vi "Main.vi"() -> ()   [LabVIEW 2014]
uses:
  vis/Controls/OtherSpec.ctl
  <vilib>/userdefined/High Color/IMAQdx.ctl
  vis/ModelEditSubVIs/ModeEditeControl.ctl
  vis/ModelEditSubVIs/ModelInfo.ctl
  vis/Controls/XYPos.ctl
  vis/Controls/MsgAction.ctl
  vis/SaveTestDataSubVI/SaveTestDataAction.ctl
  vis/Controls/Cam1QueueAction.ctl
  vis/Global.vi
  <vilib>/addons/database/Connection.llb/DB Tools Open Connec (String).vi
  <vilib>/addons/database/NI_Database_API.lvlib
panel:
  in  "调试":bool
  out "加工代码":string
  out "退出while":bool
  in  "注销":bool
  in  "写一笔轨迹":bool
  out "文件路径":path[](array[path])
  in  "Cam1拍照-二维码":bool
  in  "基本信息 2":bool
  in  "选择产品型号":u16(ring)=1
  in  "校准":bool
  out "退出Labview":bool
  out "当前零件型号":string
  out "当前零件序号":i32
  out "ModelEditInfo":T1
  in  "设置":bool
  in  "自动":bool
  in  "退出":bool
  in  "手动":bool
  in  "主控件":enum32{"自动", "手动", "设置", "校准"}(tab)
  out "线号显示":i32
  in  "切换运行模式":bool
  in  "下一根":bool
  in  "更新线号":bool
  out "扫码状态":bool
  out "产品型号":string
  out "设备ID":string
  out "数据库连接":bool
  in  "轨迹选择":u16(ring) items=["显示单根轨迹", "显示全部轨迹"]
  in  "整理坐标展示图片":bool
  in  "线号输入":i32
  in  "写入一根轨迹到PLC":bool
  in  "Cam1拍照分析-Mark2":bool
  in  "Cam1实时":bool
  in  "相机2图片路径":path
  in  "相机1图片路径":path
  out "1#结果":bool=TRUE
  in  "Cam1拍照分析-Mark1":bool
  out "消息显示":string
  out "相机1连线":bool
  out "PLC通讯":bool
  out "IO卡连接":bool
  out "当前线号布线轨迹示意图":T3(plugin-control)
  out "上相机":T3(plugin-control)
  out "载具码":string
  out "产品编码":string
  out "操作员":string
  out "产量":cluster{i32[], i32[]}(graph)
  out "单机运行":bool
  out "线总数":dbl
  in  "手动扫码触发":bool
  out "触发上升沿":T4
  in  "IO输出":T5
  out "IO输入":T6
  out "扫码内容":string
  out "扫码状态":bool
  in  "打开表格":bool
  in  "本地路径选择":path
  in  "加载本地文件":bool
  in  "是否打开":bool
  in  "保存设置":bool
  in  "其它规格":T7={"其它勾选类规格"={"保存图片"=TRUE, "上传设备状态数据"=TRUE, "保存数据"=TRUE, "开机默认开启监控摄像头"=TRUE, "启用mark拍照 "=FALSE}, "其它数据类规格"={"相机1像素-毫米换算系数"=15.0, "相机2像素-毫米换算系数"=15.0, "D盘剩余空间预警(G)"=15.0, "视频最长录制时间(秒)"=15.0}, "相机名称"={"相机1名称"="cam1", "相机2名称"="cam1", "Cam1启用"=FALSE, "Cam2启用"=FALSE, "Basler1"=FALSE, "Basler2"=FALSE}, "参数"={"Mark1曝光时间"=500, "Mark2曝光时间"=500, "二维码曝光时间"=500}} {"其它数据类规格"."视频最长录制时间(秒)" format="%.3f"; "其它数据类规格"."D盘剩余空间预警(G)" format="%.3f"; "其它数据类规格"."相机1像素-毫米换算系数" format="%.5f"; "其它数据类规格"."相机2像素-毫米换算系数" format="%.5f"}
  out "点位信息表":string[][](table)=[["PCB1-拍照点1(Mark1)", "-73.376", "-164.238", "0.000", "-103.848", "565.620", "384.924", "377.049", "0.000", "0.000", "0.000", "0", "8", "94", "1"], ["PCB1-拍照点2(Mark2)", "-260.376", "-49.239", "0.000", "-290.450", "681.264", "384.924", "377.049", "0.000", "0.000", "0.000", "-180", "8", "94", "1"], ["拍照点3", "-73.376", "-49.239", "0.000", "-103.451", "680.618", "384.924", "377.049", "0.000", "0.000", "0.000", "0", "8", "94", "1"], ["拍照点4", "-260.376", "-164.238", "0.000", "-290.847", "566.266", "384.924", "377.049", "0.000", "0.000", "0.000", "-180", "8", "94", "1"], ["拍照点5", "-260.376", "-104.239", "0.000", "-290.640", "626.265", "384.924", "377.049", "0.000", "0.000", "0.000", "-180", "8", "94", "1"], ["拍照点6", "-240.876", "-23.738", "0.000", "-270.862", "706.698", "384.924", "377.049", "0.000", "0.000", "0.000", "90", "8", "94", "1"], ["拍照点7", "-190.876", "-23.738", "0.000", "-220.862", "706.525", "384.924", "377.049", "0.000", "0.000", "0.000", "90", "8", "94", "0"], ["拍照点8", "-142.876", "-23.738", "0.000", "-172.862", "706.359", "384.924", "377.049", "0.000", "0.000", "0.000", "90", "8", "94", "0"], ["拍照点9", "-92.876", "-23.738", "0.000", "-122.863", "706.187", "384.924", "377.049", "0.000", "0.000", "0.000", "90", "8", "94", "0"], ["拍照点10", "-73.376", "-104.239", "0.000", "-103.641", "625.619", "384.924", "377.049", "0.000", "0.000", "0.000", "0", "8", "94", "0"], ["拍照点11", "-112.876", "-169.238", "0.000", "-143.365", "560.756", "384.924", "377.049", "0.000", "0.000", "0.000", "-90", "8", "94", "0"], ["拍照点12", "-220.876", "-169.238", "0.000", "-251.364", "561.130", "384.924", "377.049", "0.000", "0.000", "0.000", "0", "8", "94", "0"], ["PCB2-拍照点1(Mark3)", "-73.376", "-164.238", "0.000", "151.457", "565.201", "384.924", "377.049", "0.000", "0.000", "-3.000", "0", "8", "94", "1"], ["PCB2-拍照点2(Mark4)", "-260.376", "-49.239", "0.000", "-35.509", "680.255", "384.924", "377.049", "0.000", "0.000", "-3.000", "-180", "8", "94", "1"], ["拍照点3", "-73.376", "-49.239", "0.000", "151.491", "680.200", "384.924", "377.049", "0.000", "0.000", "-3.000", "0", "8", "94", "1"], ["拍照点4", "-260.376", "-164.238", "0.000", "-35.543", "565.256", "384.924", "377.049", "0.000", "0.000", "-3.000", "-180", "8", "94", "1"], ["拍照点5", "-260.376", "-104.239", "0.000", "-35.525", "625.255", "384.924", "377.049", "0.000", "0.000", "-3.000", "-180", "8", "94", "1"], ["拍照点6", "-240.876", "-23.738", "0.000", "-16.001", "705.751", "384.924", "377.049", "0.000", "0.000", "-3.000", "90", "8", "94", "1"], ["拍照点7", "-190.876", "-23.738", "0.000", "33.999", "705.736", "384.924", "377.049", "0.000", "0.000", "0.000", "90", "8", "94", "0"], ["拍照点8", "-142.876", "-23.738", "0.000", "81.999", "705.722", "384.924", "377.049", "0.000", "0.000", "0.000", "90", "8", "94", "0"], ["拍照点9", "-92.876", "-23.738", "0.000", "131.999", "705.707", "384.924", "377.049", "0.000", "0.000", "0.000", "90", "8", "94", "0"], ["拍照点10", "-73.376", "-104.239", "0.000", "151.475", "625.200", "384.924", "377.049", "0.000", "0.000", "0.000", "0", "8", "94", "0"], ["拍照点11", "-112.876", "-169.238", "0.000", "111.956", "560.213", "384.924", "377.049", "0.000", "0.000", "0.000", "-90", "8", "94", "0"], ["拍照点12", "-220.876", "-169.238", "0.000", "3.956", "560.245", "384.924", "377.049", "0.000", "0.000", "0.000", "0", "8", "94", "0"]]
  out "添加的路径 2":path
  out "基本信息":T12
  out "布线前甩线":string[][](table)
  out "布线点位":string[][](table)
  out "布线后甩线":string[][](table)
  out "基本信息写入":dbl[](array[numeric])
  out "进出线编码":cluster{"进线编码":i32, "出线编码":i32}[](array[cluster])
  out "布线索引":i32
  in  "补偿值":T15={"甩线补偿值"={"下边"=23.0, "距离上边"=10.0, "左边"=7.2, "右边"=25.8}, "补偿甩线坐标偏移"={"X"=40.0, "Y"=70.0}, "mark点补偿"={"X"=-48.38, "Y"=-84.85}, "出线补偿值"=25.8, "mark规格"={"X下限"=-48.38, "X上限"=-84.85, "Y下限"=0.0, "Y 上限"=0.0, "angle下限"=0.0, "angle上限"=0.0}} {"mark规格"."angle上限" format="%#.3f"; "mark规格"."angle下限" format="%#.3f"; "mark规格"."Y下限" format="%#.3f"; "mark规格"."X下限" format="%#.3f"; "mark点补偿"."X" format="%#.3f"; "补偿甩线坐标偏移"."X" format="%#.3f"}
  in  "保存值":bool
  out "mark Angle":dbl
  out "mark1偏移":T13={"X"=0.0, "Y"=70.0} {"X" format="%#.3f"}
  in  "3-计算相机与出线口偏移量":bool
  in  "校准1-相机1拍照Mark1":bool
  in  "校准1-相机1拍照Mark2":bool
  in  "4 保存校准参数":bool
  # "光背板自动布线设备"
  # "相机1 手眼校准"
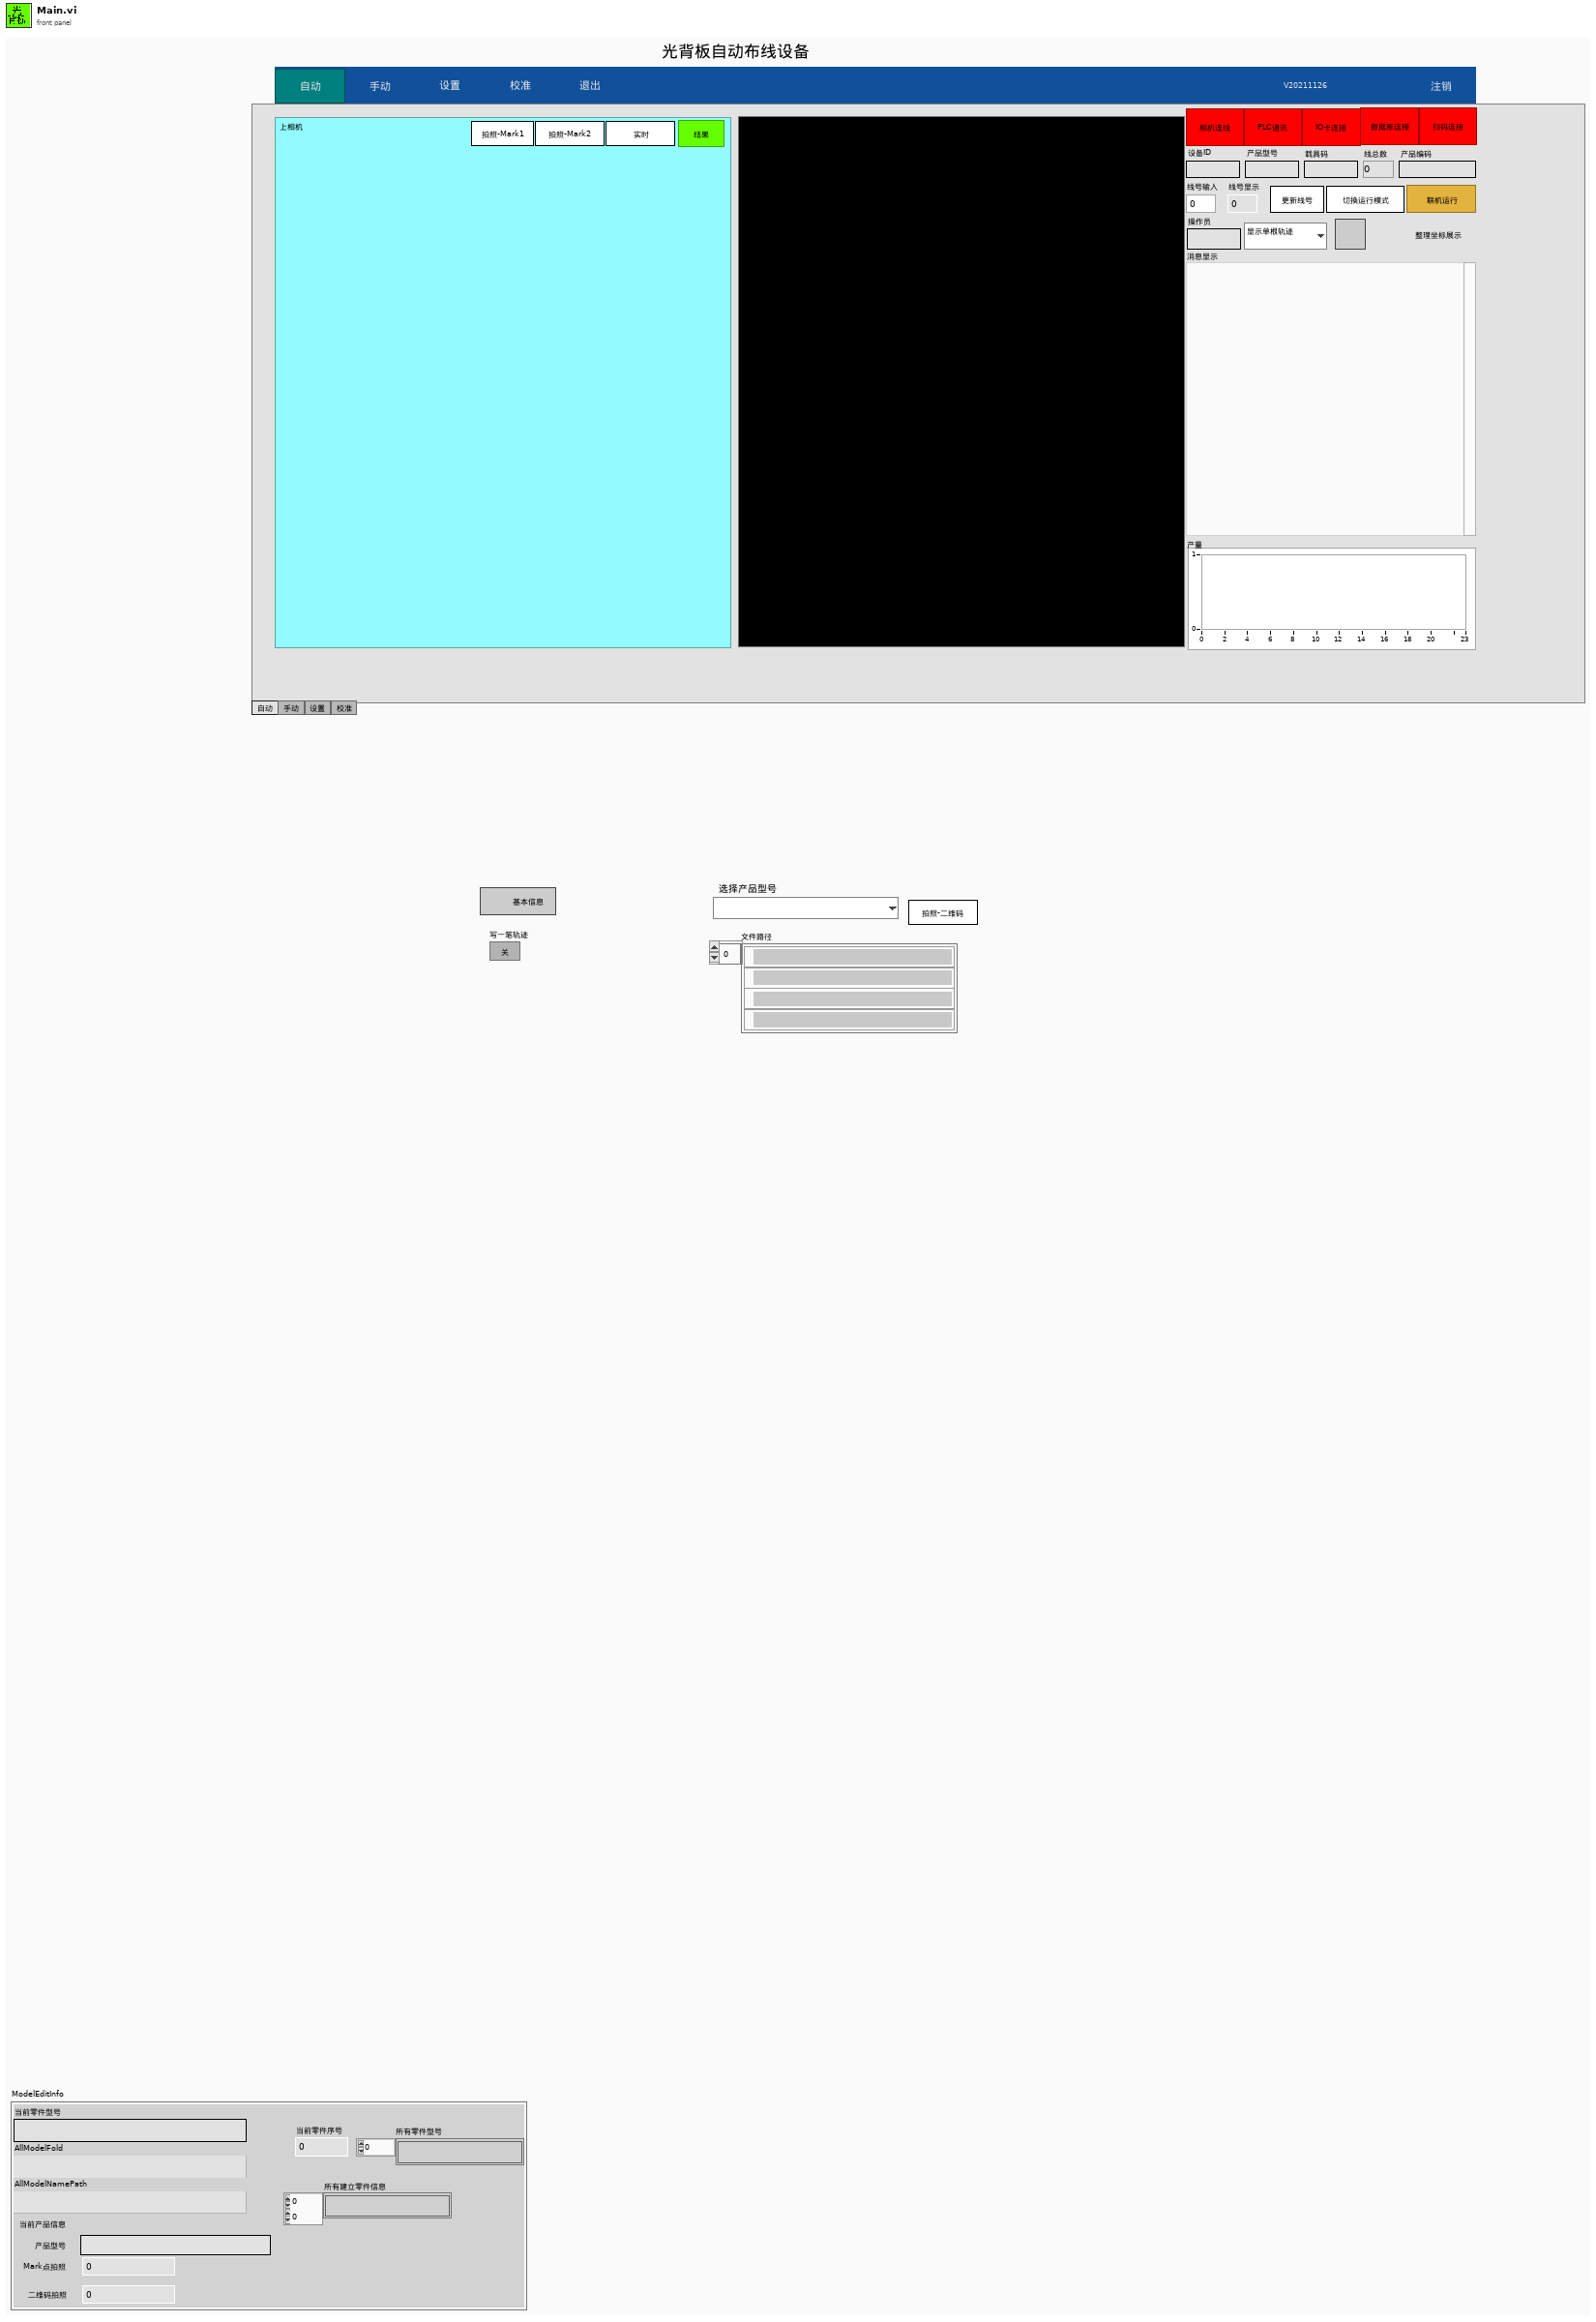
[diagram p1: front panel]
types:
  T1 = typedef "ModeEditeControl.ctl" = cluster{"AllModelFold":path, "AllModelNamePath":path, "所有零件型号":string[], "当前零件型号":string, "所有建立零件信息":string[][], "当前零件序号":i32, "当前产品信息":T2}
  T2 = typedef "ModelInfo.ctl" = cluster{"产品型号":string, "二维码拍照":u32, "Mark点拍照":u32}
  T3 = typedef "IMAQ Image.ctl" = refnum<image>
  T4 = typedef "触发上升沿.ctl" = cluster{"0 触发拍照Mark1":bool, "1 触发拍照Mark2":bool, "2 布线完成触发":bool, "3 触发扫码":bool, "4 要线信号":bool, "5 写FID":bool}
  T5 = typedef "IOoutput.ctl" = cluster{"0 返回成功信号":bool, "1 返回失败信号":bool, "2 生命信号":bool, "3 开光源":bool, "4 预留":bool, "5 预留":bool, "6 预留":bool, "7 预留":bool, "8 预留":bool, "9 预留":bool, "10 预留":bool, "11 预留":bool, "12 预留":bool, "13 预留":bool, "14 预留":bool, "15 预留":bool}
  T6 = typedef "IOinput.ctl" = cluster{"0 触发拍照Mark1":bool, "1 触发拍照Mark2":bool, "2 布线完成":bool, "3 触发扫码":bool, "4 要线信号":bool, "5 写FID":bool, "6 PLC自动运行":bool, "7 预留":bool, "8 预留":bool, "9 预留":bool, "10 预留":bool, "11 预留":bool, "12 预留":bool, "13 预留":bool, "14 预留":bool, "15预留":bool}
  T7 = typedef "OtherSpec.ctl" = cluster{"其它勾选类规格":T8, "其它数据类规格":T9, "相机名称":T10, "参数":cluster{"Mark1曝光时间":i32, "Mark2曝光时间":i32, "二维码曝光时间":i32}}
  T8 = typedef "其它勾选类规格.ctl" = cluster{"保存图片":bool, "上传设备状态数据":bool, "保存数据":bool, "开机默认开启监控摄像头":bool, "启用mark拍照 ":bool}
  T9 = typedef "其他数据类规格.ctl" = cluster{"相机1像素-毫米换算系数":dbl, "相机2像素-毫米换算系数":dbl, "D盘剩余空间预警(G)":dbl, "视频最长录制时间(秒)":dbl}
  T10 = typedef "相机名称品牌使用状态.ctl" = cluster{"相机1名称":T11, "相机2名称":T11, "Cam1启用":bool, "Cam2启用":bool, "Basler1":bool, "Basler2":bool}
  T11 = typedef "IMAQdx.ctl" = refnum<k21>
  T12 = typedef "基本信息.ctl" = cluster{"序号":dbl, "线总数":dbl, "布线板长":dbl, "布线板宽":dbl, "Mark1X":dbl, "Mark1Y":dbl, "Mark2X":dbl, "Mark2Y":dbl, "1阶段线数":dbl[], "2阶段线数":dbl[], "3阶段线数":dbl[]}
  T13 = typedef "XYPos.ctl" = cluster{"X":dbl, "Y":dbl}
  T14 = typedef "mark规格.ctl" = cluster{"X下限":dbl, "X上限":dbl, "Y下限":dbl, "Y 上限":dbl, "angle下限":dbl, "angle上限":dbl}
  T15 = cluster{"甩线补偿值":cluster{"下边":dbl, "距离上边":dbl, "左边":dbl, "右边":dbl}, "补偿甩线坐标偏移":T13, "mark点补偿":T13, "出线补偿值":dbl, "mark规格":T14}
  T16 = typedef "初始化步骤控件.ctl" = enum16{"路径&控件初始化", "界面显示初始化", "IO卡初始化", "运行模式", "选择产品型号，读取参数", "下发供料信息&Mark拍照点信息给PLC", "查询磁盘剩余空间", "结束"}
  T17 = enum32{"Invalid", "Standard", "Closed", "Hidden", "Minimized", "Maximized"}
  T18 = typedef "MsgAction.ctl" = enum16{"初始化", "添加消息", "区分结果添加消息", "清空消息", "获取消息"}
  T19 = typedef "升立德IOAction.ctl" = enum16{"IO卡初始化", "读信号(16bit)", "写信号(16bit)", "开光源", "写成功/失败信号ON", "写成功&&失败信号OFF", "写失败信号ON", "写失败信号OFF", "写生命信号", "GetInfo", "清除目标"}
  T20 = enum8{"Enabled", "Disabled", "Disabled and Grayed Out"}
  T21 = typedef "SaveTestDataAction.ctl" = enum16{"初始化", "更新机种规格", "读取表格", "第N次拍照数据写入表格(缓存)", "Mark点拍照数据存档", "取料拍螺帽数据存档", "复锁拍螺帽数据存档", "关闭表格", "打开表格"}
  T22 = typedef "控件-Excel读写选项.ctl" = enum16{"打开表格", "新增sheet", "读取sheet指定位置数据", "读取sheet整个数据", "写入sheet整个数据", "写表头", "数据存到本机", "表格是否开启状态", "关闭表格"}
  T23 = typedef "欧姆龙PLC Action.ctl" = enum16{"读设备状态", "初始化", "待命", "重新初始化", "读触发信息", "读第1组Mark点坐标", "读第2组Mark点坐标", "写基本信息", "写第1组Mark点坐标", "写第2组Mark点坐标", "写相机中心到出线头的距离", "写一笔轨迹到PLC", "写入进线前段点位", "写入板内布线点位", "写入出线布线点位", "写入数据写入完成信号", "获取信息", "写入进出线方向", "写加工信号"}
  T24 = typedef "Cam1QueueAction.ctl" = enum16{"Cam1初始化", "Cam1更新曝光时间-拍Mark点1", "Cam1更新曝光时间-拍Mark点2", "Cam1更新曝光时间-拍照二维码", "Cam1待命", "Cam1实时-Mark", "Cam1实时-二维码", "Cam1手动:Mark1", "Cam1手动:Mark2", "Cam1手动:二维码", "Cam1自动:Mark1", "Cam1自动:Mark2"}
  T25 = typedef "控件-选择相机和拍照对象.ctl" = enum16{"相机1拍Mark1", "相机1拍Mark2", "相机1拍二维码", "相机2"}
  T26 = typedef "控件-拍照PCB孔分类.ctl" = enum16{"存储校准时影像", "拍照孔-Mark1", "拍照孔-Mark2", "拍照二维码", "计算补偿量"}
  T27 = cluster{"Cam1队列":refnum<queue>, "RemoteDB":refnum<queue>, "PLC队列":refnum<queue>}
  T28 = cluster{"Value":string, "Value":string, "线号显示":i32}
  T29 = typedef "NI_Database_API.lvlib/Conn ObjectReference.ctl" = refnum<k1>
  T30 = typedef "控件-显示锁附结果动作.ctl" = enum16{"初始化锁附结果示意图", "更新当前点位锁附结果", "更新当前PCB和点位序号"}
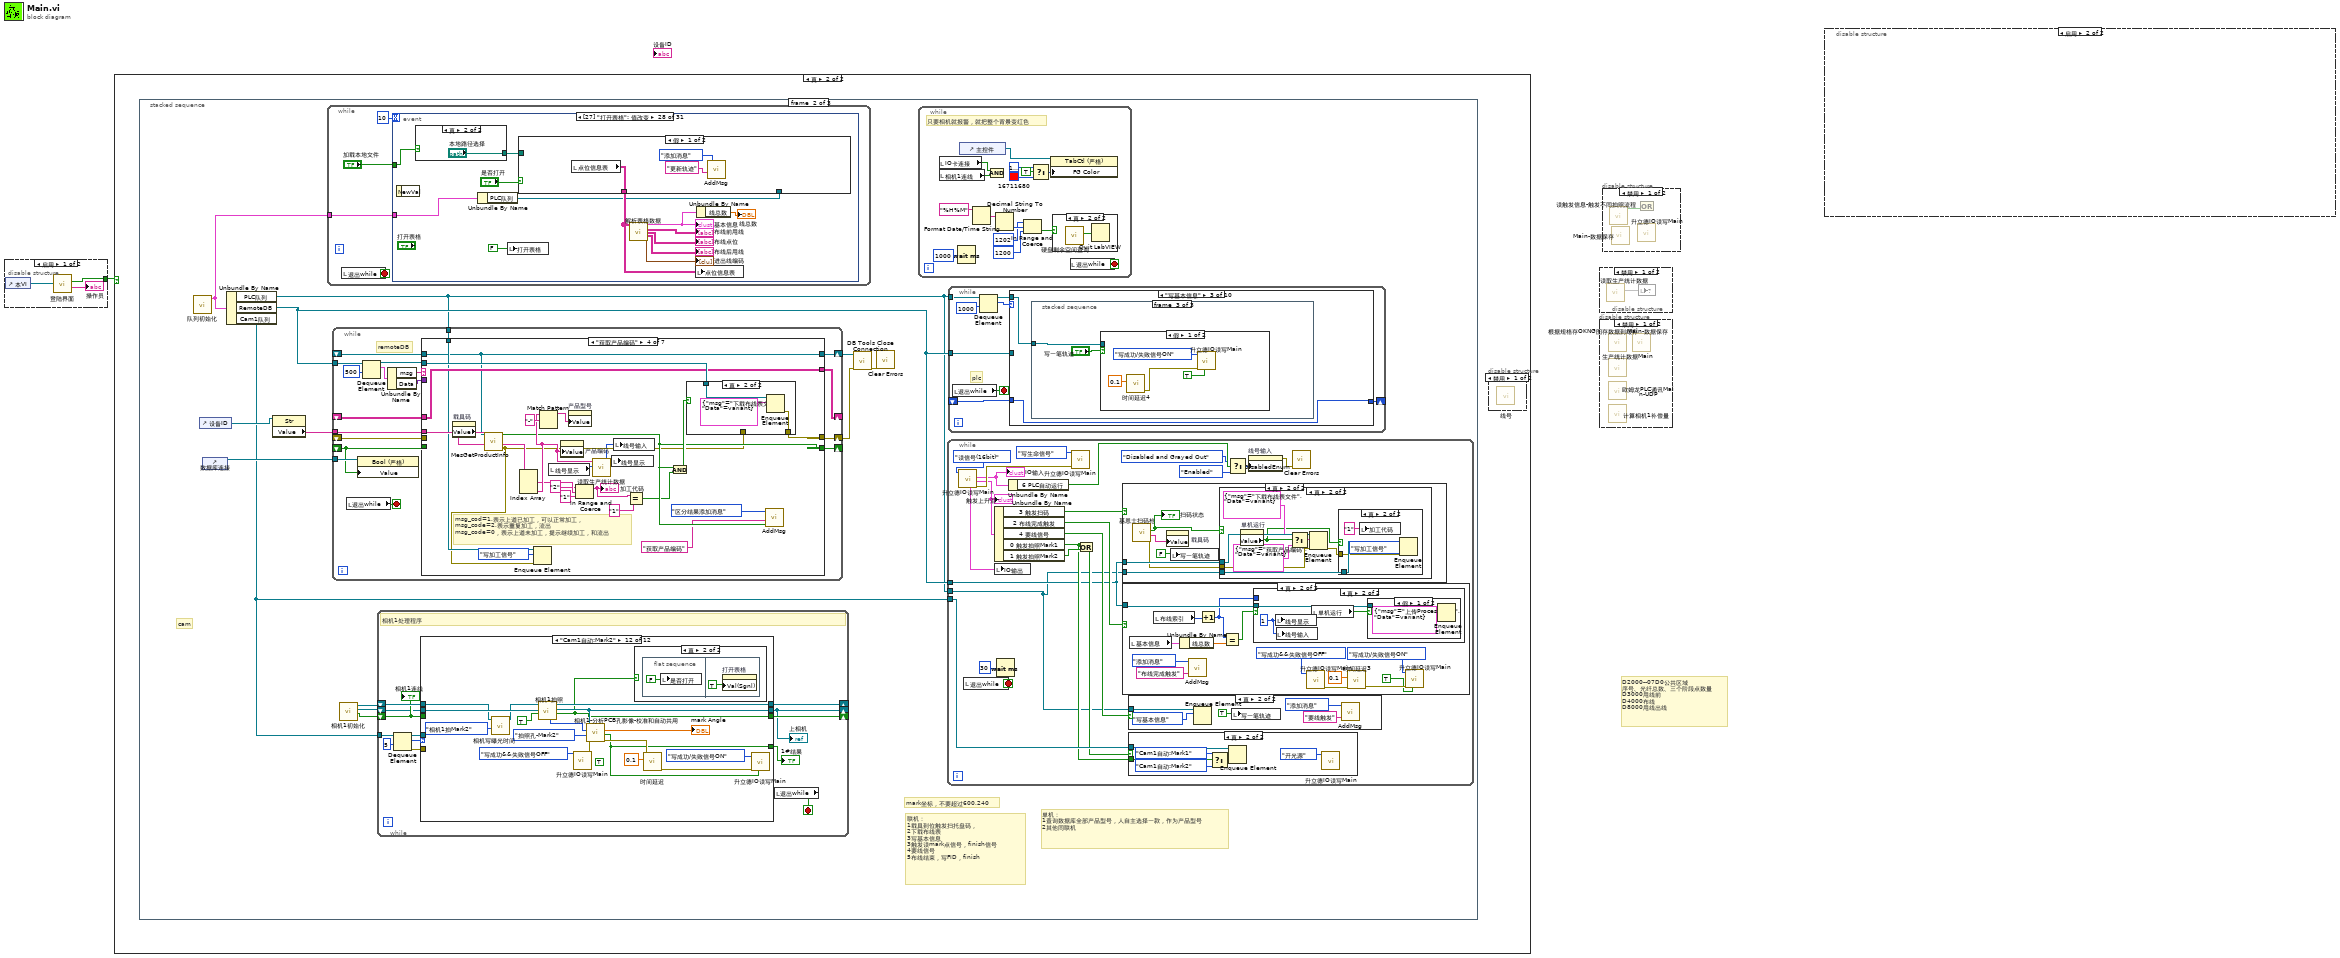
[diagram p0: block diagram]
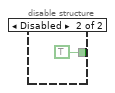
[diagram p2: hidden frame]
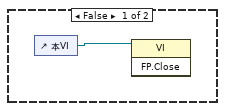
[diagram p3: hidden frame]
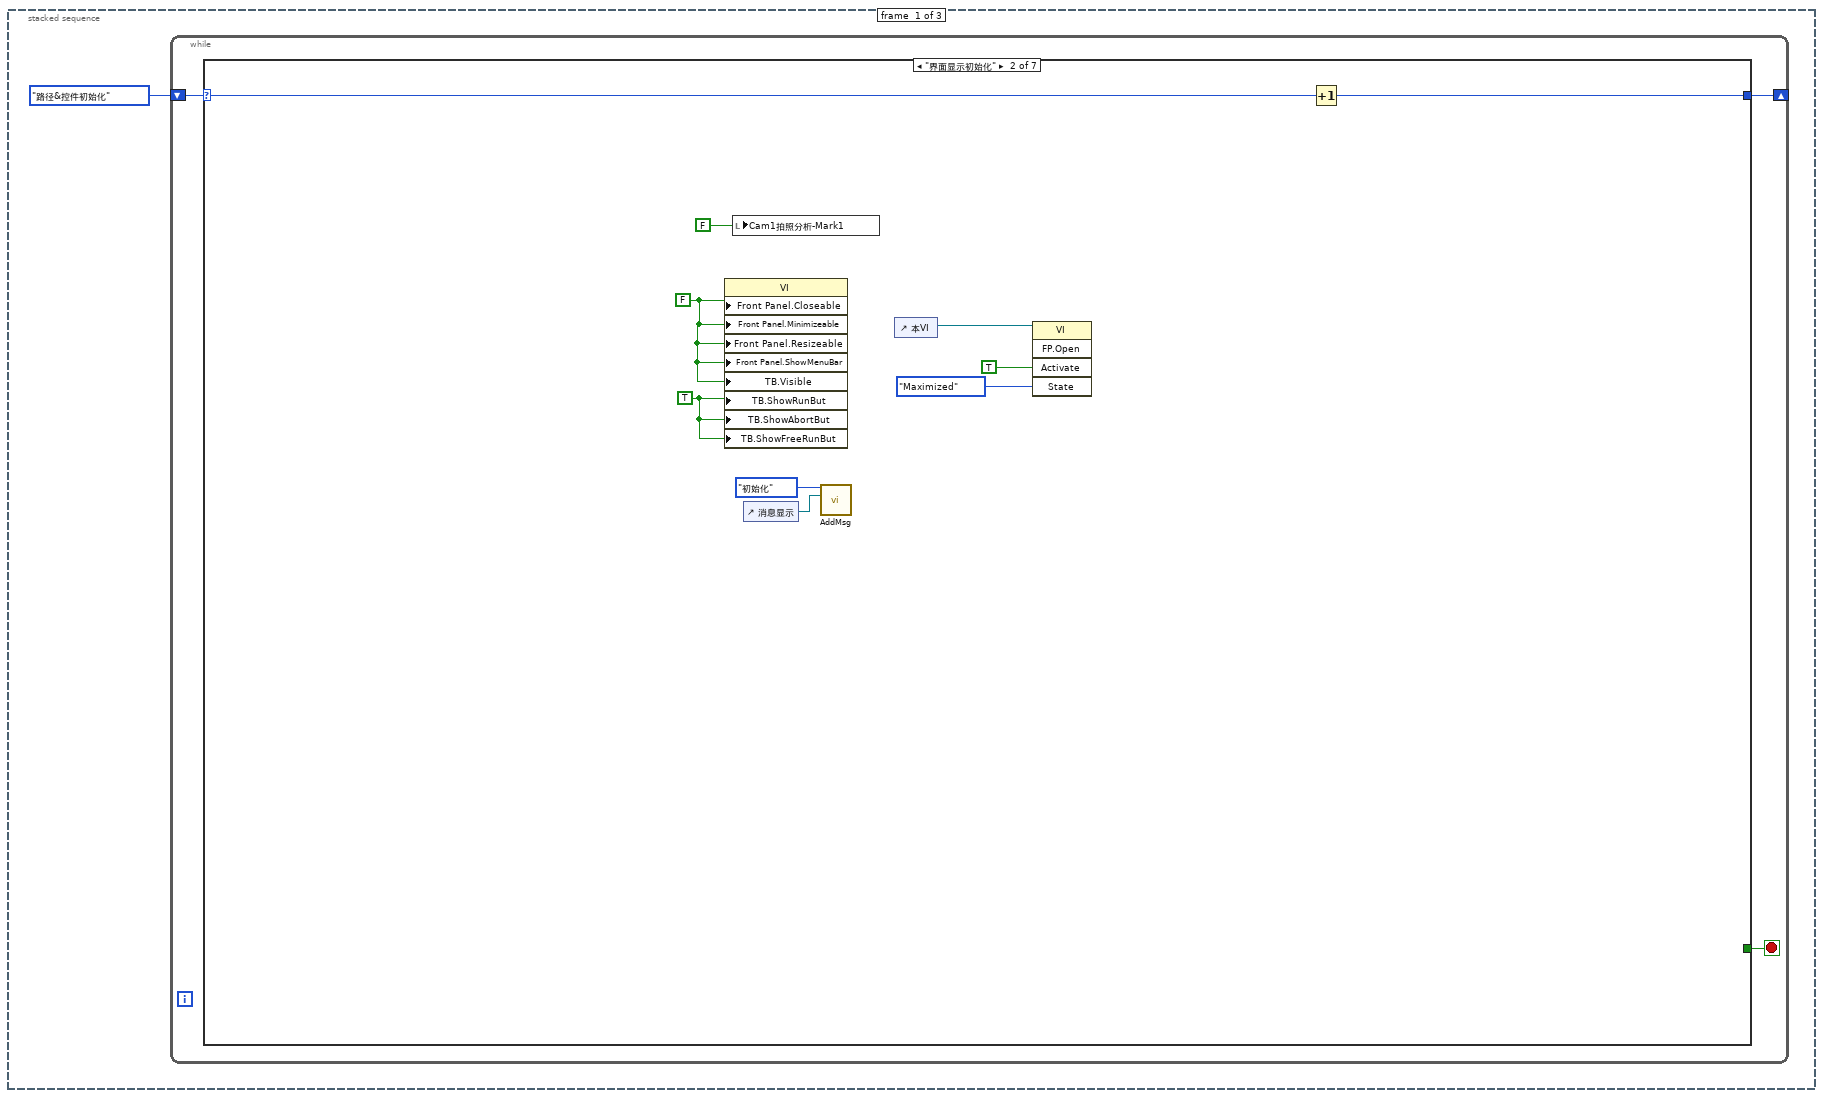
[diagram p4: hidden frame]
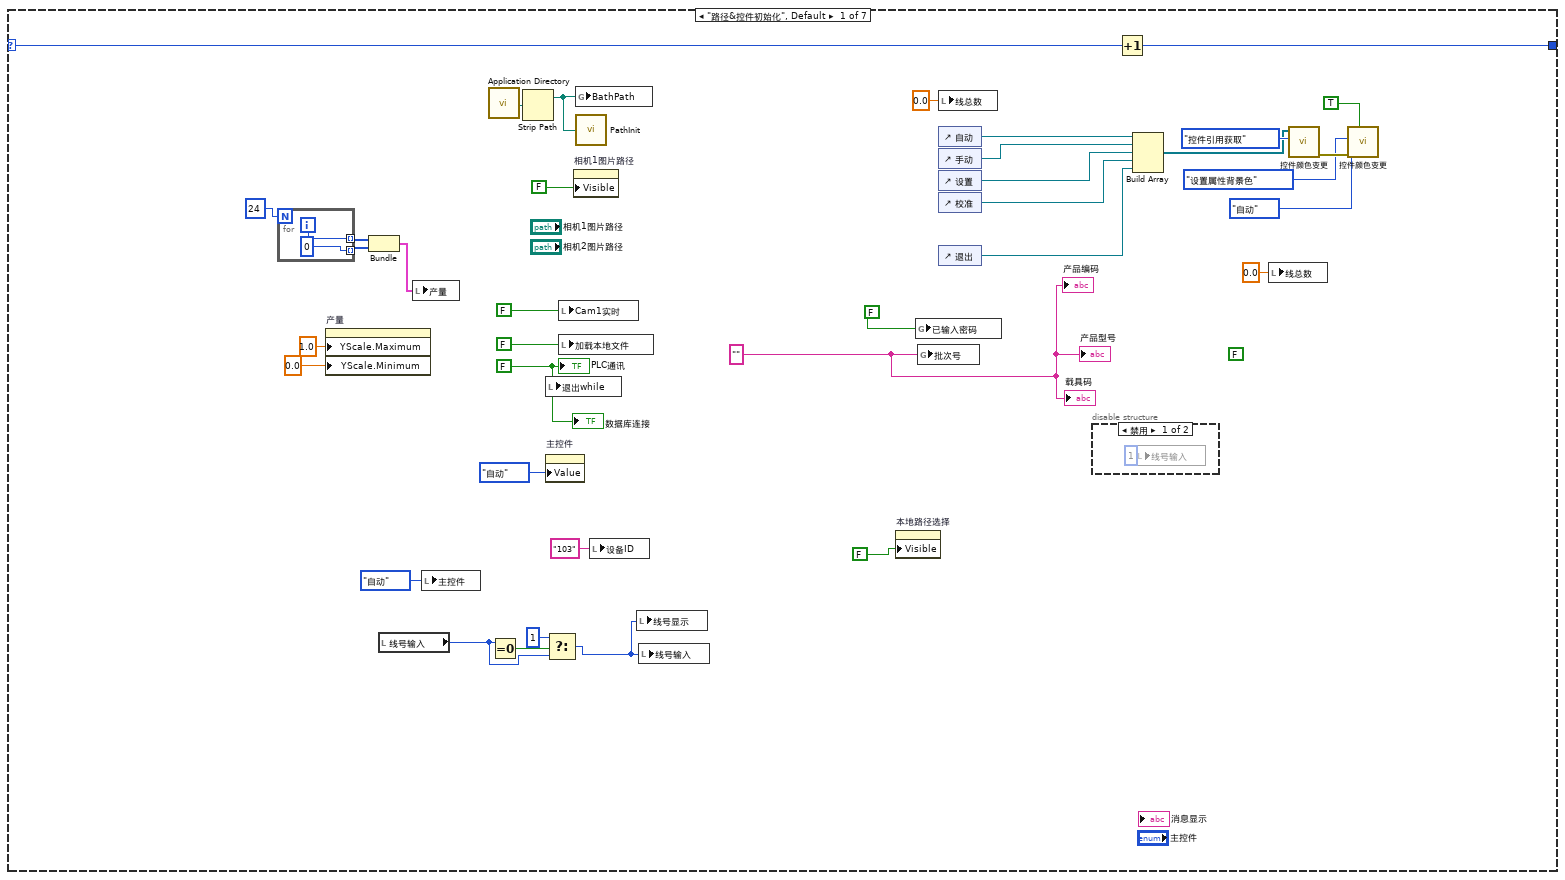
[diagram p5: hidden frame]
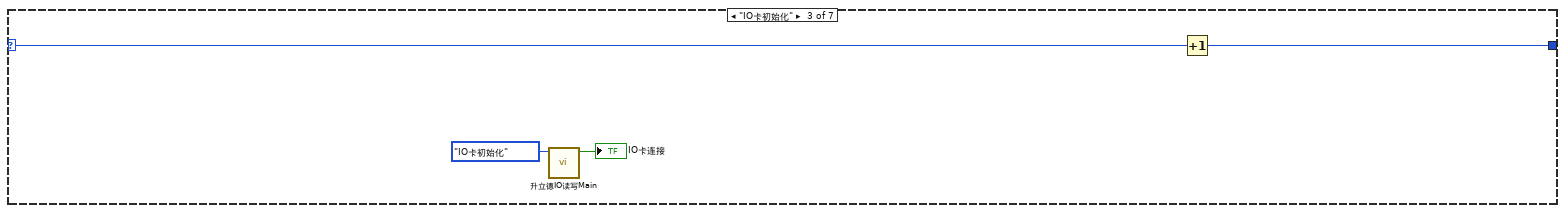
[diagram p7: hidden frame]
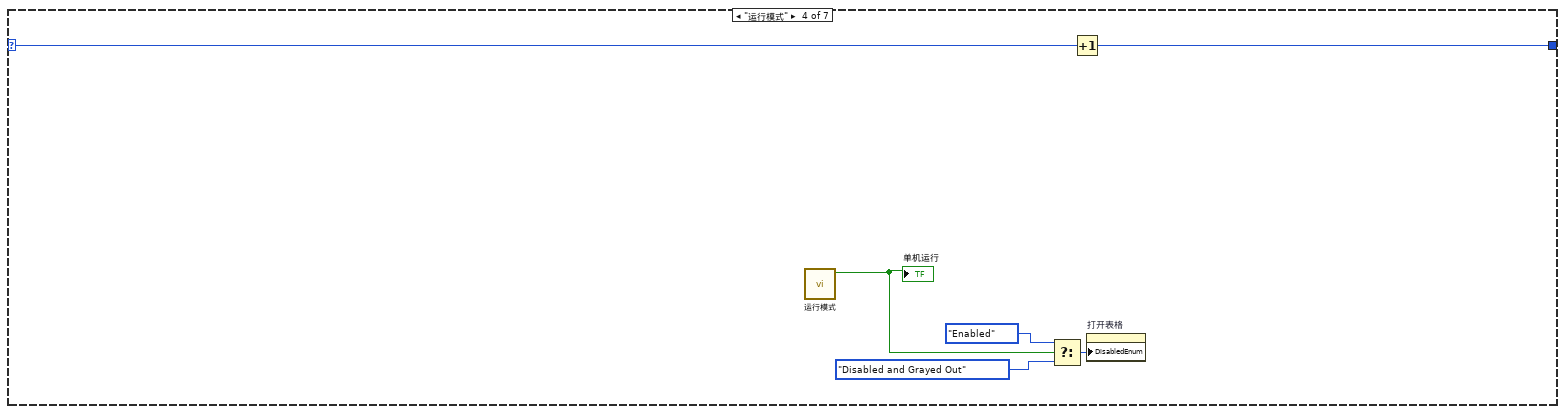
[diagram p8: hidden frame]
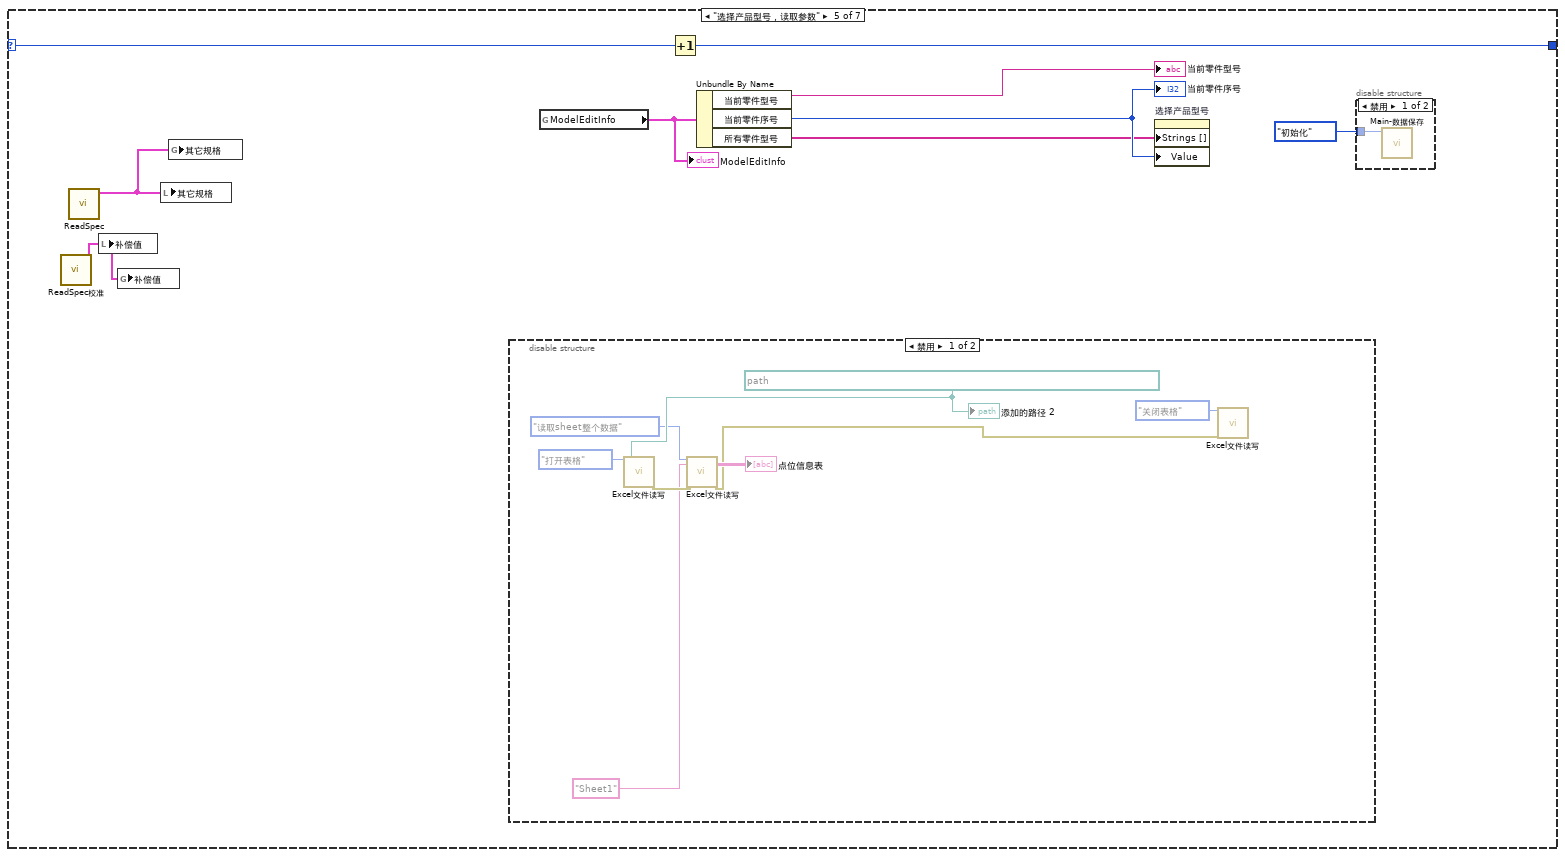
[diagram p9: hidden frame]
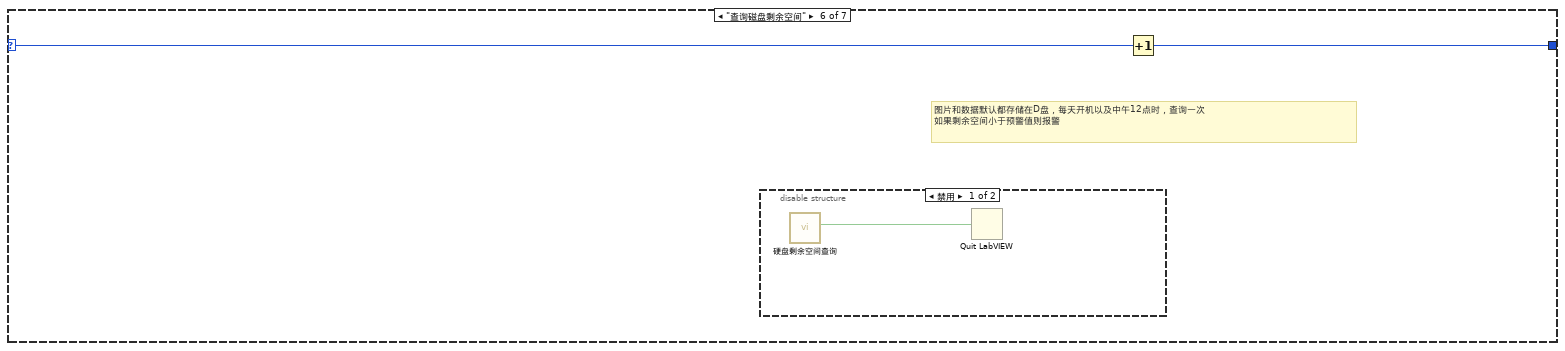
[diagram p12: hidden frame]
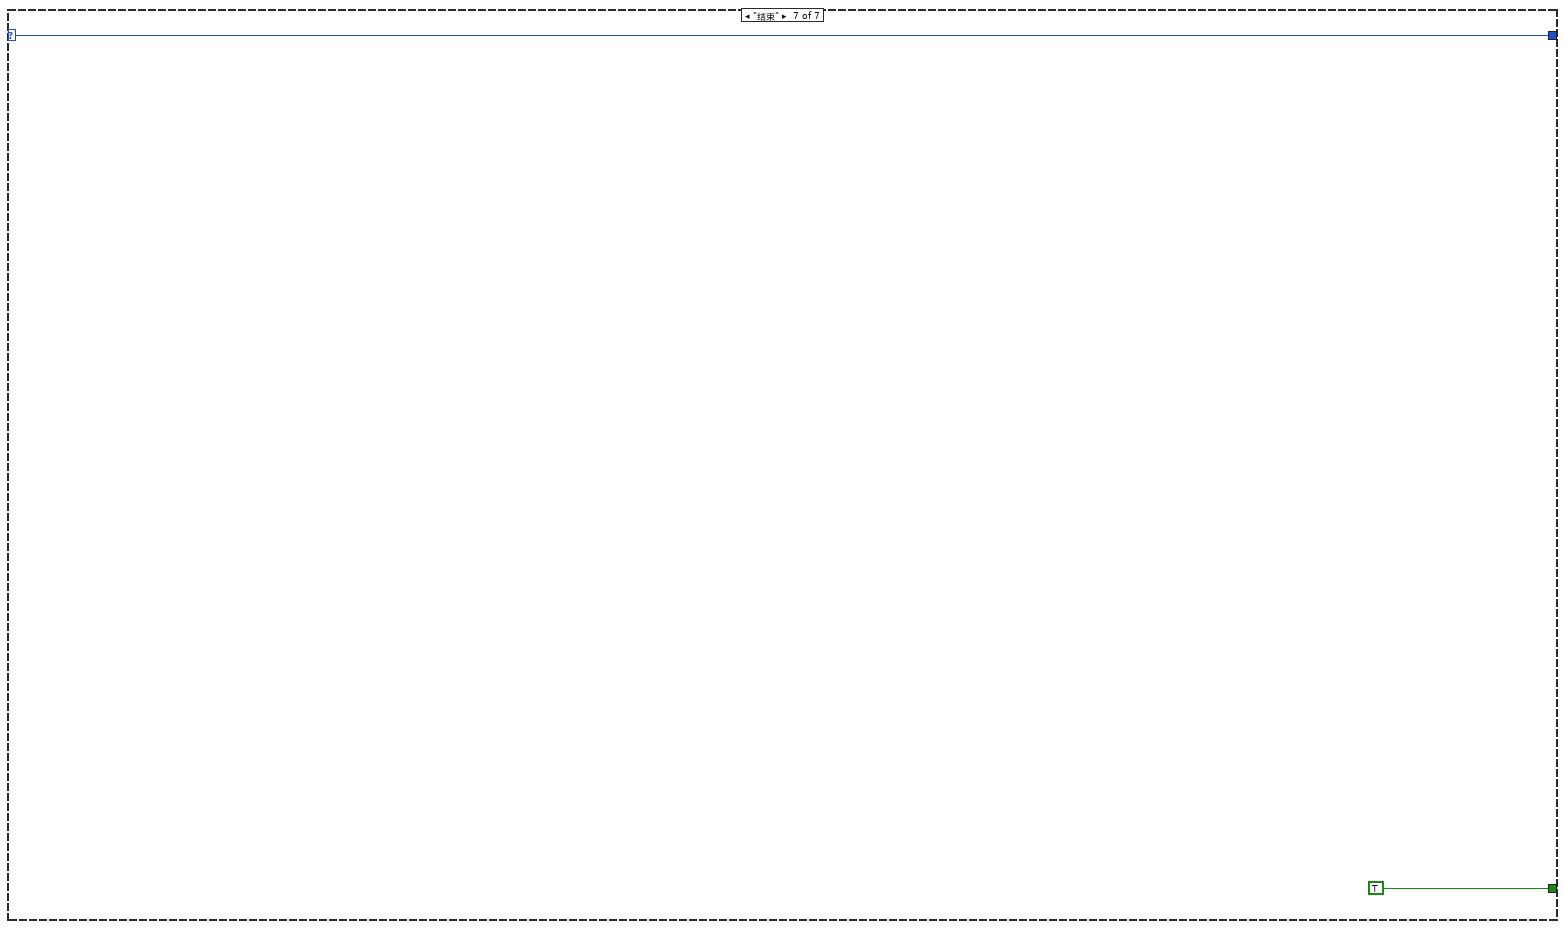
[diagram p14: hidden frame]
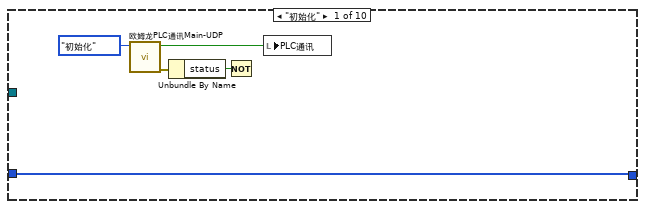
[diagram p15: hidden frame]
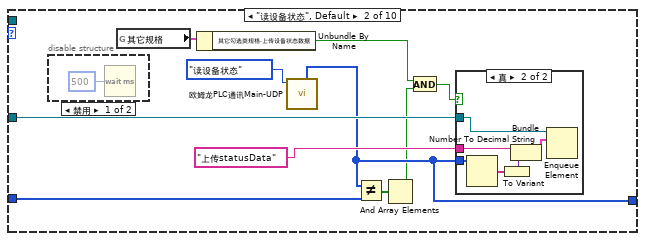
[diagram p16: hidden frame]
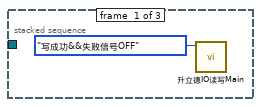
[diagram p19: hidden frame]
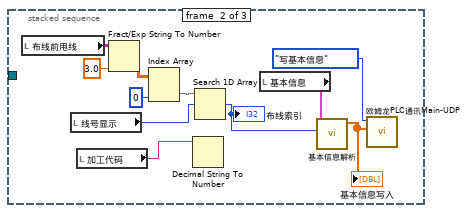
[diagram p20: hidden frame]
diagram:
  # "D2000--07D0公共区域\n序号、光纤总数、三个阶段点数量\nD3000甩线前\nD4000布线\nD8000甩线出线"
  n1 = disable-structure shown="启用" {
    disable-tunnel: [w2 TRUE ("登陆状态")] -> w1
    frame Enabled {
      n2 = control-ref of="本VI"() -> (w3:refnum<vi>)
      n3 = call "登陆界面.vi"("引用"=w3) -> ("用户名"=→"操作员":string, "登陆状态"=w2:bool)  [unwired: 9 in]
    }
    frame Disabled {
    }
  }
  n4 = case shown="真" w1 {
    frame False {
      n5 = control-ref of="本VI"() -> (w6:refnum<vi>)
      n6 = invoke class="VI" method="FP.Close"(reference=w6) -> ()  [unwired: 2 in, 3 out]
    }
    frame True {
      n7 = stacked-sequence {
        frame #0 {
          n8 = while {
            shift-right: [w9] -> _
            shift-left: 初始化步骤控件."路径&控件初始化" -> [w10]
            stop <- w8 stop-if-true
            n9 = case shown="\"界面显示初始化\"" w10 {
              selector: w10 -> [w45 w60 w62 w70 w79 w90 w93]
              tunnel: [w44 w59 w61 w69 w78 w89 w93] -> w9
              tunnel: [_ _ _ _ _ _ TRUE] -> w8
              frame "路径&控件初始化", Default {
                (unwired) FALSE ("闪烁")
                w24 = FALSE
                w21 = "" ("批次号")
                n10 = for {
                  N: 24 -> [_]
                  tunnel: [0 ("f")] -> w14 mode=indexing
                  tunnel: [w49] -> w13 mode=indexing
                  i -> [w49]
                }
                n11 = property on="产量" class="XYGraph (严格)"("YScale.Maximum"=1.0 ("Y标尺.范围:最大值"), "YScale.Minimum"=0.0 ("Y标尺.范围:最小值")) -> ()  [unwired: 2 in, 2 out]
                n12 = Bundle(w13, w14) -> (w15:cluster{i32[], i32[]})  [unwired: 1 in]
                n13 = local read "线号输入"() -> (w27:i32)
                n14 = local write "产量"(w15) -> ()
                n15 = local write "主控件"(enum32{"自动", "手动", "设置"}."自动" ("选项卡控件")) -> ()
                n16 = call <vilib>:"Application Directory.vi"() -> ("Application Directory"=w46:path)
                n17 = Equal To 0?(x=w27) -> (x = 0?=w29:bool)
                n18 = Strip Path(path=w46) -> (stripped path=w47:path)  [unwired: 1 out]
                n19 = local write "退出while"(w24) -> ()
                n20 = property on="主控件" class="TabCtl (严格)"("Value"=enum32{"自动", "手动", "设置"}."自动" ("主选项卡")) -> ()  [unwired: 2 in, 2 out]
                n21 = Select(t=1, s=w29, f=w27) -> (s? t:f=w16:i32)
                n22 = local write "Cam1实时"(FALSE ("Cam1实时-拍PCB孔")) -> ()
                n23 = local write "加载本地文件"(FALSE ("在线拍照模式/加载图片分析")) -> ()
                n24 = property on="相机1图片路径" class="Path"("Visible"=FALSE ("可见")) -> ()  [unwired: 2 in, 2 out]
                n25 = global write "Global.vi" "BathPath"(w47) -> ()
                n26 = call "PathInit.vi"("基路径"=w47) -> ()
                n27 = local write "设备ID"("103" ("设备ID")) -> ()
                n28 = local write "线号显示"(w16) -> ()
                n29 = local write "线号输入"(w16) -> ()
                n30 = property on="本地路径选择" class="Path"("Visible"=FALSE ("可见")) -> ()  [unwired: 2 in, 2 out]
                n31 = global write "Global.vi" "已输入密码"(FALSE ("已输入密码")) -> ()
                n32 = global write "Global.vi" "批次号"(w21) -> ()
                n33 = local write "线总数"(0.0 ("线总数")) -> ()
                n34 = control-ref of="自动"() -> (w32:refnum<vi>)
                n35 = control-ref of="手动"() -> (w33:refnum<vi>)
                n36 = control-ref of="设置"() -> (w34:refnum<vi>)
                n37 = control-ref of="校准"() -> (w35:refnum<vi>)
                n38 = control-ref of="退出"() -> (w36:refnum<vi>)
                n39 = disable-structure shown="禁用" {
                  frame Disabled {
                    n40 = local write "线号输入"(1 ("线号")) -> ()
                  }
                  frame Enabled {
                  }
                }
                n41 = Increment(x=w45) -> (x+1=w44:T16)
                n42 = Build Array(w32, w33, w34, w35, w36) -> (w37:refnum<vi>[])
                n43 = local write "线总数"(0.0 ("线总数")) -> ()
                n44 = call "控件颜色变更.vi"("选项"=enum16{"控件引用获取", "设置属性背景色", "还原所有背景色"}."控件引用获取", "引用"=w37) -> ("error out"=w31:errorcluster)  [unwired: 8 in, 1 out]
                n45 = call "控件颜色变更.vi"("更新"=TRUE, "error in (no error)"=w31, "控件选择"=enum16{"自动", "手动", "设置", "校准", "退出"}."自动", "选项"=enum16{"控件引用获取", "设置属性背景色", "还原所有背景色"}."设置属性背景色") -> ()  [unwired: 6 in, 2 out]
                "PLC通讯" <- w24
                "数据库连接" <- w24
                "载具码" <- w21
                "产品型号" <- w21
                "产品编码" <- w21
              }
              frame "界面显示初始化" {
                w55 = TRUE ("工具栏:显示运行按钮")
                w54 = FALSE ("前面板窗口:可关闭")
                n46 = property class="VI"("Front Panel.Closeable"=w54, "Front Panel.Minimizeable"=w54, "Front Panel.Resizeable"=w54, "Front Panel.ShowMenuBar"=w54, "TB.Visible"=w54, "TB.ShowRunBut"=w55, "TB.ShowAbortBut"=w55, "TB.ShowFreeRunBut"=w55) -> ()  [unwired: 2 in, 2 out]
                n47 = local write "Cam1拍照分析-Mark1"(FALSE ("Cam1实时")) -> ()
                n48 = control-ref of="消息显示"() -> (w57:refnum<vi>)
                n49 = call "AddMsg.vi"("消息显示引用"=w57, "消息Action"=MsgAction."初始化") -> ()  [unwired: 2 in, 1 out]
                n50 = control-ref of="本VI"() -> (w53:refnum<vi>)
                n51 = invoke class="VI" method="FP.Open"(reference=w53, "Activate"=TRUE ("激活？"), "State"=T17."Maximized" ("状态")) -> ()  [unwired: 2 in, 5 out]
                n52 = Increment(x=w60) -> (x+1=w59:T16)
              }
              frame "IO卡初始化" {
                n53 = call "升立德IO读写Main.vi"("选项"=升立德IOAction."IO卡初始化") -> ("结果"=→"IO卡连接":bool)  [unwired: 6 in, 4 out]
                n54 = Increment(x=w62) -> (x+1=w61:T16)
              }
              frame "运行模式" {
                n55 = call "运行模式.vi"() -> ("单机运行"=w68:bool)  [unwired: 10 in]
                "单机运行" <- w68
                n56 = Select(t=T20."Enabled" ("禁用"), s=w68, f=T20."Disabled and Grayed Out" ("禁用")) -> (s? t:f=w67:T20)
                n57 = Increment(x=w70) -> (x+1=w69:T16)
                n58 = property on="打开表格" class="Bool (严格)"("DisabledEnum"=w67) -> ()  [unwired: 2 in, 2 out]
              }
              frame "选择产品型号，读取参数" {
                n59 = call "ReadSpec校准.vi"() -> ("补偿值"=w71:T15)  [unwired: 11 in]
                n60 = call "ReadSpec.vi"() -> ("其它规格"=w72:T7)  [unwired: 11 in]
                n61 = local write "补偿值"(w71) -> ()
                n62 = global write "Global.vi" "补偿值"(w71) -> ()
                n63 = local write "其它规格"(w72) -> ()
                n64 = global write "Global.vi" "其它规格"(w72) -> ()
                n65 = disable-structure shown="禁用" {
                  frame Disabled {
                    w86 = path "E:/光背板布线设备-20201201/最新案例480路V2-筛选例子V2测试输出.xlsx" ("file path (dialog if empty)")
                    n66 = call "Excel文件读写.vi"("选项"=控件-Excel读写选项."打开表格", "Path"=w86) -> ("error out"=w85:errorcluster)  [unwired: 15 in, 2 out]
                    n67 = call "Excel文件读写.vi"("选项"=控件-Excel读写选项."读取sheet整个数据", "sheet name"="Sheet1", "error in"=w85) -> ("data"=→"点位信息表":string[][], "error out"=w81:errorcluster)  [unwired: 14 in, 1 out]
                    n68 = call "Excel文件读写.vi"("选项"=控件-Excel读写选项."关闭表格", "error in"=w81) -> ()  [unwired: 15 in, 3 out]
                    "添加的路径 2" <- w86
                  }
                  frame Enabled {
                  }
                }
                n69 = global read "Global.vi" "ModelEditInfo"() -> (w73:T1)
                "ModelEditInfo" <- w73
                n70 = Increment(x=w79) -> (x+1=w78:T16)
                n71 = Unbundle By Name(w73) -> ("当前零件型号"=→"当前零件型号":string, "当前零件序号"=w77:i32, "所有零件型号"=w76:string[])
                "当前零件序号" <- w77
                n72 = property on="选择产品型号" class="Ring (严格)"("Strings []"=w76, "Value"=w77) -> ()  [unwired: 2 in, 2 out]
                n73 = disable-structure shown="禁用" {
                  disable-tunnel: SaveTestDataAction."初始化" ("选项") -> [w88 _]
                  frame Disabled {
                    n74 = call "Main-数据保存.vi"("选项"=w88) -> ()  [unwired: 8 in, 1 out]
                  }
                  frame Enabled {
                  }
                }
              }
              frame "查询磁盘剩余空间" {
                # "图片和数据默认都存储在D盘，每天开机以及中午12点时，查询一次\n如果剩余空间小于预警值则报警"
                n75 = disable-structure shown="禁用" {
                  frame Disabled {
                    n76 = call "硬盘剩余空间查询.vi"() -> ("磁盘剩余空间不够"=w91:bool)  [unwired: 7 in, 2 out]
                    n77 = Quit LabVIEW(quit? (T)=w91) -> ()
                  }
                  frame Enabled {
                  }
                }
                n78 = Increment(x=w90) -> (x+1=w89:T16)
              }
              frame "结束" {
              }
            }
          }
        }
        frame #1 {
          # "mark坐标，不要超过600,240"
          # "单机：\n1查询数据库全部产品型号，人自主选择一款，作为产品型号\n2其他同联机"
          # "联机：\n1载具到位触发扫托盘码，\n2下载布线表 \n3写基本信息\n3触发读mark点信号，finish信号\n4要线信号\n5布线结束，写FID，finish"
          # "cam"
          n79 = call "队列初始化.vi"() -> ("输出队列"=w103:T27)  [unwired: 11 in]
          n80 = control-ref of="设备ID"() -> (w98:refnum<vi>)
          n81 = control-ref of="数据库连接"() -> (w101:refnum<vi>)
          n82 = Unbundle By Name(w103) -> ("PLC队列"=w95:refnum<queue>, "RemoteDB"=w96:refnum<queue>, "Cam1队列"=w94:refnum<queue>)
          n83 = property class="Str"(reference=w98) -> ("Value"=w97:string)  [unwired: 1 in, 2 out]
          n84 = while {
            tunnel: w103 -> [w644]
            stop <- w647 stop-if-true
            n85 = local read "退出while"() -> (w647:bool)
            n86 = event shown="[27] \"打开表格\": 值改变" {
              selector: _ -> [_ _ _ _ _ _ _ _ _ _ _ _ _ _ _ _ _ _ _ _ _ _ _ _ _ _ _ _ _ _ _]
              dyn-events: _ -> [_ _ _ _ _ _ _ _ _ _ _ _ _ _ _ _ _ _ _ _ _ _ _ _ _ _ _ _ _ _ _]
              timeout: 10 -> [_ _ _ _ _ _ _ _ _ _ _ _ _ _ _ _ _ _ _ _ _ _ _ _ _ _ _ _ _ _ _]
              tunnel: "加载本地文件" -> [_ _ _ _ _ _ _ _ _ _ _ _ _ _ _ _ w754 w773 _ _ _ _ _ _ _ _ _ w843 _ _ _]
              tunnel: w644 -> [_ _ _ _ _ _ _ w690 _ _ _ _ _ _ _ w747 w753 w772 w791 _ _ _ _ w817 w823 _ _ w842 w867 w873 w876]
              event Timeout {
                n87 = event-data() -> ()  [unwired: 1 in, 3 out]
                n88 = global read "Global.vi" "登陆状态"() -> (w655:cluster{"用户名称":string, "用户权限":string})
                n89 = Unbundle By Name(w655) -> ("用户权限"=w651:string)
                n90 = control-ref of="下一根"() -> (w648:refnum<vi>)
                n91 = control-ref of="设置"() -> (w653:refnum<vi>)
                n92 = control-ref of="校准"() -> (w654:refnum<vi>)
                n93 = Equal?(x=w651, y="技术员") -> (x = y?=w649:bool)
                n94 = Build Array(w653, w654, w648) -> (w652:refnum<vi>[])
                n95 = for {
                  tunnel: w652 -> [w657] mode=indexing
                  tunnel: w649 -> [w656]
                  n96 = case shown="真" w656 {
                    tunnel: w657 -> [w658 w660]
                    frame False {
                      n97 = property class="Bool (严格)"(reference=w658, "Visible"=FALSE ("可见")) -> ()  [unwired: 1 in, 2 out]
                    }
                    frame True {
                      n98 = property class="Bool (严格)"(reference=w660, "Visible"=TRUE ("可见")) -> ()  [unwired: 1 in, 2 out]
                    }
                  }
                }
              }
              event "保存设置": Mouse Up {
                n99 = event-data() -> ()  [unwired: 1 in, 1 out]
                n100 = flat-sequence {
                  frame #0 {
                    n101 = call "SaveSpec.vi"("其它规格"="其它规格") -> ()  [unwired: 3 in, 1 out]
                  }
                  frame #1 {
                    n102 = call "ReadSpec.vi"() -> ("其它规格"=w663:T7)  [unwired: 11 in]
                    n103 = global write "Global.vi" "其它规格"(w663) -> ()
                    n104 = local write "其它规格"(w663) -> ()
                  }
                }
              }
              event "保存值": Value Change {
                n105 = event-data() -> ("NewVal"=w664:bool)  [unwired: 1 in]
                n106 = case shown="真" w664 {
                  frame False {
                  }
                  frame True {
                    n107 = flat-sequence {
                      frame #0 {
                        n108 = call "Save校准Spec.vi"("补偿值"="补偿值") -> ()  [unwired: 4 in]
                      }
                      frame #1 {
                        n109 = call "ReadSpec校准.vi"() -> ("补偿值"=w666:T15)  [unwired: 11 in]
                        n110 = local write "补偿值"(w666) -> ()
                        n111 = global write "Global.vi" "补偿值"(w666) -> ()
                      }
                    }
                  }
                }
              }
              event "手动": Value Change {
                n112 = event-data() -> ("NewVal"=w667:bool)  [unwired: 1 in]
                n113 = case shown="真" w667 {
                  frame False {
                  }
                  frame True {
                    n114 = control-ref of="主控件"() -> (w673:refnum<vi>)
                    n115 = call "隐藏页面.vi"("主选项卡"=enum32{"自动", "手动", "设置"}."手动", "TabControl输入"=w673) -> ()
                    n116 = local write "手动"(FALSE ("手动")) -> ()
                    n117 = call "控件颜色变更.vi"("更新"=TRUE, "控件选择"=enum16{"自动", "手动", "设置", "校准", "退出"}."手动", "选项"=enum16{"控件引用获取", "设置属性背景色", "还原所有背景色"}."设置属性背景色") -> ()  [unwired: 7 in, 2 out]
                  }
                }
              }
              event "手动扫码触发": Value Change {
                n118 = event-data() -> ("NewVal"=w674:bool)  [unwired: 1 in]
                n119 = case shown="真" w674 {
                  frame False {
                  }
                  frame True {
                    n120 = call "基恩士扫码枪.vi"() -> ("扫码内容"=→"扫码内容":string, "扫码成功"=→"扫码状态":bool)  [unwired: 9 in, 1 out]
                  }
                }
              }
              event "更新线号": Value Change {
                n121 = event-data() -> ("NewVal"=w677:bool)  [unwired: 1 in]
                n122 = case shown="真" w677 {
                  frame False {
                  }
                  frame True {
                    n123 = call "输入密码对话框.vi"() -> ("密码正确"=w678:bool)  [unwired: 11 in]
                    n124 = case shown="真" w678 {
                      frame False {
                      }
                      frame True {
                        "线号显示" <- "线号输入"
                      }
                    }
                  }
                }
              }
              event "下一根": Value Change {
                n125 = event-data() -> ("NewVal"=w680:bool)  [unwired: 1 in]
                n126 = case shown="真" w680 {
                  frame False {
                  }
                  frame True {
                    n127 = local read "基本信息"() -> (w685:T12)
                    n128 = local read "线号输入"() -> (w684:i32)
                    n129 = Unbundle By Name(w685) -> ("线总数"=w683:dbl)
                    n130 = Equal?(x=w684, y=w683) -> (x = y?=w682:bool)
                    n131 = case shown="假" w682 {
                      tunnel: [w687 1] -> w681
                      tunnel: w684 -> [w686 _]
                      frame False {
                        n132 = Increment(x=w686) -> (x+1=w687:i32)
                      }
                      frame True {
                      }
                    }
                    n133 = local write "线号显示"(w681) -> ()
                    n134 = local write "线号输入"(w681) -> ()
                  }
                }
              }
              event "切换运行模式": Value Change {
                n135 = event-data() -> ("NewVal"=w691:bool)  [unwired: 1 in]
                n136 = Unbundle By Name(w690) -> ("RemoteDB"=w689:refnum<queue>)
                n137 = case shown="真" w691 {
                  tunnel: w689 -> [_ w692]
                  frame False {
                  }
                  frame True {
                    n138 = call "输入密码对话框.vi"() -> ("密码正确"=w693:bool)  [unwired: 11 in]
                    n139 = case shown="真" w693 {
                      tunnel: w692 -> [_ w694]
                      frame False {
                      }
                      frame True {
                        n140 = local read "单机运行"() -> (w696:bool)
                        n141 = Not(x=w696) -> (.not. x?=w695:bool)
                        n142 = local write "单机运行"(w695) -> ()
                        n143 = case shown="真" w695 {
                          tunnel: w694 -> [_ w698]
                          frame False {
                          }
                          frame True {
                            n144 = Enqueue Element(queue=w698, element=cluster{"msg":string, "Data":variant} {"msg"="获取数据库All产品型号", "Data"=variant} ("元素")) -> ()  [unwired: 2 in, 3 out]
                          }
                        }
                      }
                    }
                  }
                }
              }
              event "自动": Value Change {
                n145 = event-data() -> ("NewVal"=w699:bool)  [unwired: 1 in]
                n146 = case shown="真" w699 {
                  frame False {
                  }
                  frame True {
                    n147 = control-ref of="主控件"() -> (w705:refnum<vi>)
                    n148 = local write "自动"(FALSE ("手动")) -> ()
                    n149 = call "隐藏页面.vi"("主选项卡"=enum32{"自动", "手动", "设置"}."自动", "TabControl输入"=w705) -> ()
                    n150 = call "控件颜色变更.vi"("更新"=TRUE, "控件选择"=enum16{"自动", "手动", "设置", "校准", "退出"}."自动", "选项"=enum16{"控件引用获取", "设置属性背景色", "还原所有背景色"}."设置属性背景色") -> ()  [unwired: 7 in, 2 out]
                  }
                }
              }
              event "退出": Value Change {
                n151 = event-data() -> ("NewVal"=w706:bool)  [unwired: 1 in]
                n152 = case shown="真" w706 {
                  frame False {
                  }
                  frame True {
                    n153 = local read "线号显示"() -> (w710:i32)
                    n154 = property on="产品编码" class="Str"() -> ("Value"=w711:string)  [unwired: 2 in, 2 out]
                    n155 = property on="载具码" class="Str"() -> ("Value"=w712:string)  [unwired: 2 in, 2 out]
                    n156 = Bundle("Value"=w712, "Value"=w711, "线号显示"=w710) -> (w709:T28)  [unwired: 1 in]
                    n157 = call "close_labview.vi"("输入簇"=w709) -> ("退出while"=→"退出while":bool, "退出Labview"=w708:bool)
                    "退出Labview" <- w708
                    n158 = call "控件颜色变更.vi"("更新"=FALSE, "控件选择"=enum16{"自动", "手动", "设置", "校准", "退出"}."退出", "选项"=enum16{"控件引用获取", "设置属性背景色", "还原所有背景色"}."设置属性背景色") -> ("控件"=w714:i32)  [unwired: 7 in, 1 out]
                    n159 = call "控件颜色变更.vi"("更新"=w708, "控件选择"=w714, "选项"=enum16{"控件引用获取", "设置属性背景色", "还原所有背景色"}."设置属性背景色") -> ()  [unwired: 7 in, 2 out]
                  }
                }
              }
              event "调试": Value Change {
                n160 = event-data() -> ()  [unwired: 1 in, 6 out]
                n161 = local write "调试"(FALSE ("调试")) -> ()
                n162 = call "输入密码对话框.vi"() -> ("密码正确"=w718:bool)  [unwired: 11 in]
                n163 = case shown="真" w718 {
                  frame False {
                  }
                  frame True {
                    n164 = local write "退出while"(TRUE ("退出while")) -> ()
                    n165 = local write "退出Labview"(FALSE ("退出Labview")) -> ()
                  }
                }
              }
              event "设置": Value Change {
                n166 = event-data() -> ("NewVal"=w722:bool)  [unwired: 1 in]
                n167 = case shown="真" w722 {
                  frame False {
                  }
                  frame True {
                    n168 = control-ref of="主控件"() -> (w727:refnum<vi>)
                    n169 = call "隐藏页面.vi"("主选项卡"=enum32{"自动", "手动", "设置"}."设置", "TabControl输入"=w727) -> ()
                    n170 = local write "设置"(FALSE ("手动")) -> ()
                    n171 = call "控件颜色变更.vi"("控件选择"=enum16{"自动", "手动", "设置", "校准", "退出"}."设置", "选项"=enum16{"控件引用获取", "设置属性背景色", "还原所有背景色"}."设置属性背景色") -> ()  [unwired: 8 in, 2 out]
                  }
                }
              }
              event "注销": Value Change {
                n172 = event-data() -> ()  [unwired: 1 in, 1 out]
                n173 = control-ref of="本VI"() -> (w730:refnum<vi>)
                n174 = Two Button Dialog(message="是否要注销当前登录账户" ("消息")) -> (T button?=w728:bool)  [unwired: 2 in]
                n175 = case shown="真" w728 {
                  tunnel: w730 -> [_ w732]
                  frame False {
                  }
                  frame True {
                    n176 = call "登陆界面.vi"("引用"=w732) -> ("用户名"=w731:string, "登陆状态"=w733:bool)  [unwired: 9 in]
                    n177 = case shown="假" w733 {
                      tunnel: w732 -> [_ w736]
                      tunnel: w731 -> [_ w735]
                      frame False {
                        w734 = TRUE ("退出")
                        n178 = local write "退出while"(w734) -> ()
                        n179 = local write "退出Labview"(w734) -> ()
                      }
                      frame True {
                        n180 = property on="操作员" class="Str"("Value"=w735) -> ()  [unwired: 2 in, 2 out]
                        n181 = invoke class="VI" method="FP.Open"(reference=w736, "Activate"=TRUE ("激活？"), "State"=T17."Standard" ("状态")) -> ()  [unwired: 2 in, 5 out]
                      }
                    }
                  }
                }
              }
              event "校准": Value Change {
                n182 = event-data() -> ("NewVal"=w739:bool)  [unwired: 1 in]
                n183 = case shown="真" w739 {
                  frame False {
                  }
                  frame True {
                    n184 = control-ref of="主控件"() -> (w744:refnum<vi>)
                    n185 = call "隐藏页面.vi"("主选项卡"=enum32{"自动", "手动", "设置", "校准"}."校准", "TabControl输入"=w744) -> ()
                    n186 = local write "校准"(FALSE ("手动")) -> ()
                    n187 = call "控件颜色变更.vi"("控件选择"=enum16{"自动", "手动", "设置", "校准", "退出"}."校准", "选项"=enum16{"控件引用获取", "设置属性背景色", "还原所有背景色"}."设置属性背景色") -> ()  [unwired: 8 in, 2 out]
                  }
                }
              }
              event "选择产品型号": Value Change {
                n188 = event-data() -> ("NewVal"=w745:u16)  [unwired: 1 in]
                n189 = property on="选择产品型号" class="Ring (严格)"() -> ("Strings []"=w746:string[])  [unwired: 2 in, 2 out]
                n190 = Index Array(array=w746, index=w745) -> ()  [unwired: 1 out]
              }
              event "Cam1实时": Value Change {
                n191 = event-data() -> ("NewVal"=w748:bool)  [unwired: 1 in]
                n192 = case shown="真" w748 {
                  tunnel: w747 -> [_ w752]
                  frame False {
                  }
                  frame True {
                    n193 = Unbundle By Name(w752) -> ("Cam1队列"=w751:refnum<queue>)
                    n194 = Enqueue Element(queue=w751, element=Cam1QueueAction."Cam1实时-Mark" ("元素")) -> (error out=w749:errorcluster)  [unwired: 2 in, 2 out]
                    n195 = call <vilib>:"Clear Errors.vi"("error in (no error)"=w749) -> ()  [unwired: 5 in, 2 out]
                  }
                }
              }
              event "Cam1拍照分析-Mark1": Value Change {
                n196 = event-data() -> ("NewVal"=w755:bool)  [unwired: 1 in]
                n197 = case shown="真" w755 {
                  tunnel: w753 -> [_ w759]
                  tunnel: w754 -> [_ w758]
                  frame False {
                  }
                  frame True {
                    n198 = case shown="假" w758 {
                      tunnel: w759 -> [w768 _]
                      frame False {
                        # "在线拍照测试"
                        n199 = Unbundle By Name(w768) -> ("Cam1队列"=w767:refnum<queue>)
                        n200 = call "AddMsg.vi"("添加消息"="手动触发拍照Mark1", "消息Action"=MsgAction."添加消息") -> ()  [unwired: 2 in, 1 out]
                        n201 = Enqueue Element(queue=w767, element=Cam1QueueAction."Cam1更新曝光时间-拍Mark点1" ("元素")) -> (queue out=w763:refnum<queue>, error out=w762:errorcluster)  [unwired: 2 in, 1 out]
                        n202 = Enqueue Element(queue=w763, element=Cam1QueueAction."Cam1手动:Mark1" ("元素"), error in (no error)=w762) -> (error out=w761:errorcluster)  [unwired: 1 in, 2 out]
                        n203 = call <vilib>:"Clear Errors.vi"("error in (no error)"=w761) -> ()  [unwired: 5 in, 2 out]
                      }
                      frame True {
                        # "加载图片测试"
                        n204 = disable-structure shown="禁用" {
                          frame Disabled {
                            n205 = local read "上相机"() -> (w769:T3)
                            n206 = call "相机1图像处理.vi"("Img输入"=w769) -> ("1结果"=w771:bool, "Img输出"=w770:T3)  [unwired: 7 in, 2 out]
                            n207 = local write "上相机"(w770) -> ()
                            n208 = local write "1#结果"(w771) -> ()
                          }
                          frame Enabled {
                          }
                        }
                      }
                    }
                    n209 = local write "Cam1拍照分析-Mark1"(FALSE ("拍照分析1-PCB孔")) -> ()
                    n210 = local write "Cam1实时"(FALSE ("Cam1实时-拍PCB孔")) -> ()
                  }
                }
              }
              event "Cam1拍照分析-Mark2": Value Change {
                n211 = event-data() -> ("NewVal"=w774:bool)  [unwired: 1 in]
                n212 = case shown="真" w774 {
                  tunnel: w772 -> [_ w778]
                  tunnel: w773 -> [_ w777]
                  frame False {
                  }
                  frame True {
                    n213 = case shown="假" w777 {
                      tunnel: w778 -> [w787 _]
                      frame False {
                        # "在线拍照测试"
                        n214 = Unbundle By Name(w787) -> ("Cam1队列"=w786:refnum<queue>)
                        n215 = Enqueue Element(queue=w786, element=Cam1QueueAction."Cam1更新曝光时间-拍Mark点2" ("元素")) -> (queue out=w780:refnum<queue>, error out=w782:errorcluster)  [unwired: 2 in, 1 out]
                        n216 = call "AddMsg.vi"("添加消息"="手动触发拍照Mark2", "消息Action"=MsgAction."添加消息") -> ()  [unwired: 2 in, 1 out]
                        n217 = Enqueue Element(queue=w780, element=Cam1QueueAction."Cam1手动:Mark2" ("元素"), error in (no error)=w782) -> (error out=w781:errorcluster)  [unwired: 1 in, 2 out]
                        n218 = call <vilib>:"Clear Errors.vi"("error in (no error)"=w781) -> ()  [unwired: 5 in, 2 out]
                      }
                      frame True {
                        # "加载图片测试"
                        n219 = disable-structure shown="禁用" {
                          frame Disabled {
                            n220 = local read "上相机"() -> (w788:T3)
                            n221 = call "相机1图像处理.vi"("Img输入"=w788) -> ("1结果"=w790:bool, "Img输出"=w789:T3)  [unwired: 7 in, 2 out]
                            n222 = local write "上相机"(w789) -> ()
                            n223 = local write "1#结果"(w790) -> ()
                          }
                          frame Enabled {
                          }
                        }
                      }
                    }
                    n224 = local write "Cam1拍照分析-Mark2"(FALSE ("拍照分析1-PCB孔")) -> ()
                    n225 = local write "Cam1实时"(FALSE ("Cam1实时-拍PCB孔")) -> ()
                  }
                }
              }
              event "Cam1拍照-二维码": Value Change {
                n226 = event-data() -> ("NewVal"=w792:bool)  [unwired: 1 in]
                n227 = case shown="真" w792 {
                  tunnel: w791 -> [_ w803]
                  frame False {
                  }
                  frame True {
                    # "在线拍照测试"
                    n228 = Unbundle By Name(w803) -> ("Cam1队列"=w801:refnum<queue>)
                    n229 = local write "Cam1拍照-二维码"(FALSE ("Cam1测试")) -> ()
                    n230 = call "AddMsg.vi"("添加消息"="手动触发拍照二维码", "消息Action"=MsgAction."添加消息") -> ()  [unwired: 2 in, 1 out]
                    n231 = Enqueue Element(queue=w801, element=Cam1QueueAction."Cam1更新曝光时间-拍照二维码" ("元素")) -> (queue out=w796:refnum<queue>, error out=w793:errorcluster)  [unwired: 2 in, 1 out]
                    n232 = Enqueue Element(queue=w796, element=Cam1QueueAction."Cam1手动:二维码" ("元素"), error in (no error)=w793) -> (error out=w794:errorcluster)  [unwired: 1 in, 2 out]
                    n233 = local write "Cam1实时"(FALSE ("Cam1实时-拍PCB孔")) -> ()
                    n234 = call <vilib>:"Clear Errors.vi"("error in (no error)"=w794) -> ()  [unwired: 5 in, 2 out]
                  }
                }
              }
              event "相机1图片路径": Value Change {
                n235 = event-data() -> ("NewVal"=w805:path)  [unwired: 1 in]
                n236 = call "OpenGrayImg.vi"("Image Name"="Cam1Img", "Img Path"=w805) -> ("Image Out"=w804:T3)
                n237 = local write "上相机"(w804) -> ()
              }
              event "加载本地文件": Value Change {
                n238 = event-data() -> ("NewVal"=w808:bool)  [unwired: 1 in]
                n239 = case shown="真" w808 {
                  tunnel: [FALSE ("可见") TRUE ("可见")] -> w807
                  frame False {
                  }
                  frame True {
                    n240 = local write "本地路径选择"(path "") -> ()
                  }
                }
                n241 = property on="本地路径选择" class="Path"("Visible"=w807) -> ()  [unwired: 2 in, 2 out]
              }
              event "相机2图片路径": Value Change {
                n242 = event-data() -> ("NewVal"=w813:path)  [unwired: 1 in]
                n243 = call "OpenGrayImg.vi"("Image Name"="Cam2Img", "Img Path"=w813) -> ()  [unwired: 1 out]
              }
              event Value Change {
                n244 = event-data() -> ("NewVal"=w815:T5)  [unwired: 1 in]
                n245 = call "升立德IO读写Main.vi"("IO输出"=w815, "选项"=升立德IOAction."写信号(16bit)") -> ("IO输出"=w814:T5)  [unwired: 5 in, 4 out]
                n246 = local write "IO输出"(w814) -> ()
              }
              event "校准1-相机1拍照Mark1": Value Change {
                n247 = event-data() -> ("NewVal"=w818:bool)  [unwired: 1 in]
                n248 = case shown="真" w818 {
                  tunnel: w817 -> [_ w820]
                  frame False {
                  }
                  frame True {
                    n249 = Unbundle By Name(w820) -> ("Cam1队列"=w822:refnum<queue>)
                    n250 = Enqueue Element(queue=w822, element=Cam1QueueAction."Cam1手动:Mark1" ("元素")) -> (error out=w821:errorcluster)  [unwired: 2 in, 2 out]
                    n251 = call <vilib>:"Clear Errors.vi"("error in (no error)"=w821) -> ()  [unwired: 5 in, 2 out]
                  }
                }
              }
              event "校准1-相机1拍照Mark2": Value Change {
                n252 = event-data() -> ("NewVal"=w824:bool)  [unwired: 1 in]
                n253 = case shown="真" w824 {
                  tunnel: w823 -> [_ w826]
                  frame False {
                  }
                  frame True {
                    n254 = Unbundle By Name(w826) -> ("Cam1队列"=w828:refnum<queue>)
                    n255 = Enqueue Element(queue=w828, element=Cam1QueueAction."Cam1手动:Mark2" ("元素")) -> (error out=w827:errorcluster)  [unwired: 2 in, 2 out]
                    n256 = call <vilib>:"Clear Errors.vi"("error in (no error)"=w827) -> ()  [unwired: 5 in, 2 out]
                  }
                }
              }
              event "3-计算相机与出线口偏移量": Value Change {
                n257 = event-data() -> ("NewVal"=w829:bool)  [unwired: 1 in]
                n258 = case shown="真" w829 {
                  frame False {
                  }
                  frame True {
                  }
                }
              }
              event "4 保存校准参数": Value Change {
                n259 = event-data() -> ("NewVal"=w830:bool)  [unwired: 1 in]
                n260 = case shown="真" w830 {
                  frame False {
                  }
                  frame True {
                    n261 = call "Save校准Spec.vi"() -> ()  [unwired: 5 in]
                  }
                }
              }
              event "打开表格": Value Change {
                n262 = event-data() -> ()  [unwired: 1 in, 1 out]
                n263 = case shown="真" w843 {
                  tunnel: [w864 "本地路径选择"] -> w836
                  frame False {
                    n264 = local read "文件路径"() -> (w865:path[])
                    n265 = Index Array(array=w865) -> (element=w864:path)  [unwired: 1 in]
                  }
                  frame True {
                  }
                }
                n266 = Unbundle By Name(w842) -> ("PLC队列"=w835:refnum<queue>)
                n267 = local write "打开表格"(FALSE ("打开表格")) -> ()
                n268 = case shown="假" "是否打开" {
                  tunnel: [w846 w856] -> w838
                  tunnel: w836 -> [_ w855]
                  tunnel: w835 -> [_ w850]
                  frame False {
                    n269 = local read "点位信息表"() -> (w846:string[][])
                    n270 = call "AddMsg.vi"("添加消息"="更新轨迹", "消息Action"=MsgAction."添加消息") -> ()  [unwired: 2 in, 1 out]
                  }
                  frame True {
                    n271 = call "Excel文件读写.vi"("选项"=控件-Excel读写选项."打开表格", "Path"=w855) -> ("error out"=w860:errorcluster)  [unwired: 15 in, 2 out]
                    n272 = call "Excel文件读写.vi"("选项"=控件-Excel读写选项."读取sheet整个数据", "sheet name"="", "error in"=w860) -> ("data"=w856:string[][], "error out"=w857:errorcluster)  [unwired: 14 in, 1 out]
                    n273 = call "Excel文件读写.vi"("选项"=控件-Excel读写选项."关闭表格", "error in"=w857) -> ("error out"=w853:errorcluster)  [unwired: 15 in, 2 out]
                    n274 = Unbundle By Name(w853) -> ("status"=w852:bool)
                    n275 = Not(x=w852) -> (.not. x?=w849:bool)
                    n276 = call "AddMsg.vi"("Result"=w849, "添加消息"="打开表格", "消息Action"=MsgAction."区分结果添加消息") -> ()  [unwired: 1 in, 1 out]
                    n277 = case shown="真" w849 {
                      tunnel: w850 -> [_ w863]
                      tunnel: 欧姆龙PLC_Action."写基本信息" ("元素") -> [_ w862]
                      frame False {
                      }
                      frame True {
                        n278 = Enqueue Element(queue=w863, element=w862) -> ()  [unwired: 2 in, 3 out]
                      }
                    }
                  }
                }
                n279 = call "解析表格数据.vi"("点位信息表"=w838) -> ("基本信息"=w833:T12, "布线前甩线"=→"布线前甩线":string[][], "布线点位"=→"布线点位":string[][], "布线后甩线"=→"布线后甩线":string[][], "进出线编码"=→"进出线编码":cluster{"进线编码":i32, "出线编码":i32}[])  [unwired: 10 in]
                "基本信息" <- w833
                n280 = local write "点位信息表"(w838) -> ()
                n281 = Unbundle By Name(w833) -> ("线总数"=→"线总数":dbl)
              }
              event "整理坐标展示图片": Value Change {
                n282 = event-data() -> ("NewVal"=w868:bool)  [unwired: 1 in, 2 out]
                n283 = case shown="真" w868 {
                  tunnel: w867 -> [_ w870]
                  frame False {
                  }
                  frame True {
                    n284 = Unbundle By Name(w870) -> ("PLC队列"=w869:refnum<queue>)
                    n285 = Enqueue Element(queue=w869, element=欧姆龙PLC_Action."获取信息" ("元素")) -> ()  [unwired: 2 in, 3 out]
                  }
                }
              }
              event "基本信息 2": Value Change {
                n286 = event-data() -> ()  [unwired: 1 in, 3 out]
                n287 = Unbundle By Name(w873) -> ("PLC队列"=w872:refnum<queue>)
                n288 = Enqueue Element(queue=w872, element=欧姆龙PLC_Action."写基本信息" ("元素")) -> ()  [unwired: 2 in, 3 out]
              }
              event "写入一根轨迹到PLC": Value Change {
                n289 = event-data() -> ()  [unwired: 1 in, 3 out]
                n290 = Unbundle By Name(w876) -> ("PLC队列"=w875:refnum<queue>)
                n291 = Enqueue Element(queue=w875, element=欧姆龙PLC_Action."写基本信息" ("元素")) -> ()  [unwired: 2 in, 3 out]
                n292 = call "AddMsg.vi"("Result"=TRUE, "添加消息"="手动写入一根轨迹" ("消息显示"), "消息Action"=MsgAction."添加消息") -> ()  [unwired: 1 in, 1 out]
              }
            }
          }
          n293 = while {
            tunnel: w96 -> [w254]
            shift-right: [w262] -> w102
            shift-left: _ -> [w259]
            tunnel: w101 -> [w261]
            shift-right: [w260] -> _
            shift-left: _ -> [w258]
            shift-right: [w256] -> w100
            shift-left: _ -> [w257]
            tunnel: w97 -> [w252]
            shift-right: [w250] -> _
            shift-left: _ -> [w251]
            tunnel: w95 -> [w249]
            stop <- w265 stop-if-true
            # "remoteDB"
            n294 = local read "退出while"() -> (w265:bool)
            n295 = property class="Bool (严格)"(reference=w261, "Value"=w258) -> ()  [unwired: 1 in, 2 out]
            n296 = Dequeue Element(queue=w254, timeout in ms (-1)=500 ("超时毫秒(-1)")) -> (queue out=w253:refnum<queue>, element=w264:cluster{"msg":string, "Data":variant})  [unwired: 1 in, 2 out]
            n297 = Unbundle By Name(w264) -> ("msg"=w263:string, "Data"=w255:variant)
            n298 = case shown="\"获取产品编码\"" w263 {
              tunnel: [w280 w313 w324 w336 w367 w391 w425] -> w262
              tunnel: [w277 w311 w321 w341 w360 w385 w398] -> w260
              tunnel: w259 -> [w281 _ w324 w336 w369 w388 w426]
              tunnel: w258 -> [_ _ _ _ _ _ _]
              tunnel: [w282 w310 w319 w352 w370 w387 w406] -> w256
              tunnel: w257 -> [w282 _ w323 _ _ w384 _]
              tunnel: w255 -> [_ _ _ _ _ w392 _]
              tunnel: w253 -> [_ w307 _ w353 _ _ _]
              tunnel: w252 -> [w279 _ _ w348 _ w386 w417]
              tunnel: w251 -> [w276 w309 w320 w349 w363 w383 w397]
              tunnel: [w278 w309 w320 w349 w363 w383 w397] -> w250
              tunnel: w249 -> [_ _ _ w338 _ _ _]
              frame "统计产量数据", Default {
                n299 = disable-structure shown="启用" {
                  disable-tunnel: w281 -> [w289 w290]
                  disable-tunnel: [w288 w290] -> w280
                  disable-tunnel: w279 -> [w287 _]
                  disable-tunnel: [w286 _] -> w278
                  disable-tunnel: [w285 _] -> w277
                  disable-tunnel: [w283 _] -> w267
                  frame Enabled {
                    n300 = call "MesGetALLProduct.vi"("equipment_code"=w287, "类型"="统计产量数据", "connection reference"=w289) -> ("查找的结果"=w286:string[][], "connection out"=w288:T29, "错误状态"=w285:bool, "非空"=w283:bool)  [unwired: 4 in, 1 out]
                  }
                  frame Disabled {
                  }
                }
                n301 = Array Size(array=w276) -> (size(s)=w269:i32[])
                n302 = Index Array(array=w269) -> (element=w270:i32)  [unwired: 1 in]
                n303 = Not Equal?(x=w278, y=w276) -> (x != y?=w275:bool[][])
                n304 = Equal To 0?(x=w270) -> (x = 0?=w271:bool)
                n305 = Or Array Elements(Boolean array=w275) -> (logical OR=w273:bool)
                n306 = And(x=w267, y=w271) -> (x .and. y?=w268:bool)
                n307 = Or(x=w273, y=w268) -> (x .or. y?=w272:bool)
                n308 = And(x=w267, y=w272) -> (x .and. y?=w274:bool)
                n309 = case shown="真" w274 {
                  tunnel: w278 -> [_ w293]
                  frame False {
                  }
                  frame True {
                    n310 = Decimal String To Number(string=w293) -> (number=w298:i32[][])  [unwired: 2 in, 1 out]
                    n311 = for {
                      N: 24 -> [_]
                      tunnel: [0 ("f")] -> w297 mode=indexing
                      tunnel: [w306] -> w296 mode=indexing
                      i -> [w306]
                    }
                    n312 = for {
                      tunnel: w298 -> [w303] mode=indexing
                      shift-right: [w301] -> w295
                      shift-left: w297 -> [w304]
                      tunnel: [w300] -> w294 mode=indexing
                      n313 = Index Array(array=w303) -> (element #1=w302:i32, element #2=w300:i32)  [unwired: 2 in]
                      n314 = Replace Array Subset(array=w304, new element=w300, index=w302) -> (w301:i32[])
                    }
                    n315 = Array Max & Min(array=w294) -> (max value=w291:i32)  [unwired: 3 out]
                    n316 = property on="产量" class="XYGraph (严格)"("YScale.Maximum"=w291) -> ()  [unwired: 2 in, 2 out]
                    n317 = Bundle(w296, w295) -> (→"产量":cluster{i32[], i32[]})  [unwired: 1 in]
                  }
                }
              }
              frame "Initialize" {
                n318 = call-poly <vilib>:"DB Tools Open Connection.vi"("connection information"="Provider=MSDASQL.1;Persist Security Info=False;Data Source=mes_board") -> ("error out"=w310:errorcluster, "connection reference"=w313:T29)  [unwired: 7 in]
                n319 = local read "单机运行"() -> (w308:bool)
                n320 = Unbundle By Name(w310) -> ("status"=w312:bool)
                n321 = Not(x=w312) -> (.not. x?=w311:bool)
                n322 = case shown="真" w308 {
                  tunnel: w307 -> [_ w318]
                  frame False {
                  }
                  frame True {
                    n323 = Enqueue Element(queue=w318, element=cluster{"msg":string, "Data":variant} {"msg"="获取数据库All产品型号", "Data"=variant} ("元素")) -> ()  [unwired: 2 in, 3 out]
                  }
                }
                n324 = call "AddMsg.vi"("Result"=w311, "添加消息"="数据库连接", "消息Action"=MsgAction."区分结果添加消息") -> ()  [unwired: 1 in, 1 out]
              }
              frame "下载布线表文件" {
                n325 = property on="产品型号" class="Str"() -> ("Value"=w328:string)  [unwired: 2 in, 2 out]
                n326 = call "下载图片AOI.vi"("error in (no error)"=w323, "文件类型"="布线表", "产品型号"=w328) -> ("error out"=w319:errorcluster, "获取成功"=w321:bool, "文件路径"=→"文件路径":path[])  [unwired: 5 in, 1 out]
                n327 = case shown="真" w321 {
                  frame False {
                  }
                  frame True {
                    n328 = flat-sequence {
                      frame #0 {
                        n329 = local write "是否打开"(TRUE ("是否打开")) -> ()
                      }
                      frame #1 {
                        n330 = property on="打开表格" class="Bool (严格)"("Val(Sgnl)"=TRUE ("值(信号)")) -> ()  [unwired: 2 in, 2 out]
                      }
                    }
                  }
                }
                n331 = call "AddMsg.vi"("Result"=w321, "添加消息"="下载文件", "消息Action"=MsgAction."区分结果添加消息") -> ()  [unwired: 1 in, 1 out]
              }
              frame "获取产品编码" {
                # "msg_cod=1,表示上道已加工，可以正常加工，\nmsg_code=2,表示重复加工，流出\nmsg_code=0，表示上道未加工，提示继续加工，和流出"
                n332 = property on="载具码" class="Str"() -> ("Value"=w351:string)  [unwired: 2 in, 2 out]
                n333 = call "MesGetProductInfo.vi"("设备码"=w348, "托盘编码值"=w351, "connection reference"=w336) -> ("error out"=w335:errorcluster, "加工状态"=w347:string[], "错误状态"=w341:bool)  [unwired: 6 in]
                n334 = Index Array(array=w347) -> (element #1=w345:string, element #3=w346:string)  [unwired: 3 in, 1 out]
                n335 = Enqueue Element(queue=w338, element=欧姆龙PLC_Action."写加工信号" ("元素"), error in (no error)=w335) -> ()  [unwired: 1 in, 3 out]
                n336 = Match Pattern(string=w346, regular expression="-" ("正则表达式")) -> (before substring=w350:string)  [unwired: 1 in, 3 out]
                n337 = local read "线号显示"() -> (w332:i32)
                n338 = property on="产品编码" class="Str"("Value"=w346) -> ()  [unwired: 2 in, 2 out]
                n339 = property on="产品型号" class="Str"("Value"=w350) -> ()  [unwired: 2 in, 2 out]
                n340 = In Range and Coerce(upper limit="2" ("上限"), x=w345, lower limit="1" ("下限")) -> (coerced(x)=w333:string)  [unwired: 1 out]
                "加工代码" <- w333
                n341 = call "读取生产统计数据.vi"("线号显示"=w332, "产品码"=w346) -> ("线号"=w331:i32)  [unwired: 7 in]
                n342 = local write "线号显示"(w331) -> ()
                n343 = local write "线号输入"(w331) -> ()
                n344 = Equal?(x=w333, y="1") -> (x = y?=w340:bool)
                n345 = And(x=w341, y=w340) -> (x .and. y?=w342:bool)
                n346 = case shown="真" w342 {
                  tunnel: w353 -> [_ w359]
                  tunnel: [w356 w358] -> w352
                  tunnel: w335 -> [w356 _]
                  frame False {
                  }
                  frame True {
                    n347 = Enqueue Element(queue=w359, element=cluster{"msg":string, "Data":variant} {"msg"="下载布线表文件", "Data"=variant} ("元素")) -> (error out=w358:errorcluster)  [unwired: 2 in, 2 out]
                  }
                }
                n348 = call "AddMsg.vi"("Result"=w341, "添加消息"="获取产品编码", "消息Action"=MsgAction."区分结果添加消息") -> ()  [unwired: 1 in, 1 out]
              }
              frame "获取数据库All产品型号" {
                n349 = call "MesGetALLProduct.vi"("类型"="产品型号", "connection reference"=w369) -> ("error out"=w365:errorcluster, "查找的结果"=w368:string[][], "connection out"=w367:T29, "错误状态"=w361:bool, "非空"=w362:bool)  [unwired: 5 in]
                n350 = And(x=w362, y=w361) -> (x .and. y?=w360:bool)
                n351 = case shown="真" w360 {
                  tunnel: [w373 w374] -> w370
                  tunnel: w368 -> [_ w377]
                  tunnel: w365 -> [w373 w374]
                  frame False {
                  }
                  frame True {
                    n352 = Index Array(array=w377, index (col)=0 ("禁用的索引 (列)")) -> (element=w378:string[])  [unwired: 1 in]
                    n353 = call "SelectModel.vi"("产品型号"=w378) -> ("当前零件型号"=w375:string)  [unwired: 2 in, 1 out]
                    n354 = property on="产品型号" class="Str"("Value"=w375) -> ()  [unwired: 2 in, 2 out]
                  }
                }
                n355 = local write "产品编码"("" ("product_code")) -> ()
                n356 = call "AddMsg.vi"("Result"=w360, "添加消息"="获取数据库All产品型号", "消息Action"=MsgAction."区分结果添加消息") -> ()  [unwired: 1 in, 1 out]
              }
              frame "上传statusData" {
                n357 = Variant To Data(type=string[] [] ("字段值"), Variant=w392) -> (data=w390:string[])  [unwired: 1 in, 1 out]
                n358 = Insert Into Array(array=w390, index=0 ("索引"), new element=w386) -> (w380:string[])
                n359 = Index Array(array=w380) -> (element #2=w379:string)  [unwired: 2 in, 1 out]
                n360 = call "MesProductDesc.vi"("字段值"=w380, "字段名"=string[] ["equipment_code", "equipment_status"], "error in"=w384, "table"="collect_equipment_status", "connection reference"=w388) -> ("error out"=w387:errorcluster, "connection out"=w391:T29, "错误状态"=w385:bool)  [unwired: 4 in]
                n361 = Concatenate Strings("上传status数据" ("添加消息"), w379) -> (w381:string)
                n362 = call "AddMsg.vi"("Result"=w385, "添加消息"=w381, "消息Action"=MsgAction."区分结果添加消息") -> ()  [unwired: 1 in, 1 out]
              }
              frame "上传ProcessData" {
                n363 = property on="mark1偏移" class="Clust (严格)"() -> ("Value"=w403:T13)  [unwired: 2 in, 2 out]
                n364 = property on="mark Angle" class="DigNum (严格)"() -> ("Value"=w404:dbl)  [unwired: 2 in, 2 out]
                n365 = property on="操作员" class="Str"() -> ("Value"=w420:string)  [unwired: 2 in, 2 out]
                n366 = local read "产品编码"() -> (w415:string)
                n367 = local read "载具码"() -> (w416:string)
                n368 = Unbundle(w403) -> ("X"=w402:dbl, "Y"=w401:dbl)
                n369 = Concatenate Strings("操作员" ("字符串"), ":" ("字符串"), w420, ";" ("字符串")) -> (w418:string)
                n370 = Format Date/Time String(time format string (%c)="%Y-%m-%d %H:%M:%S;" ("时间格式字符串(%c)")) -> (date/time string=w423:string)  [unwired: 2 in]
                n371 = Format Into String(format string="偏移量:%.3f,%.3f;偏移角度:%.3f;", w402, w401, w404) -> (resulting string=w405:string)  [unwired: 2 in, 1 out]
                n372 = Concatenate Strings(w405, "结束时间:" ("字符串"), w423, w418) -> (w414:string)
                n373 = Build Array(w417, w416, w415, w414) -> (w413:string[])
                n374 = call "升立德IO读写Main.vi"("选项"=升立德IOAction."写成功&&失败信号OFF") -> ("error out"=w409:errorcluster)  [unwired: 6 in, 4 out]
                n375 = call "MesProductDesc.vi"("字段值"=w413, "字段名"=string[] ["equipment_code", "pallet_code", "product_code", "process_data"], "error in"=w409, "table"="collect_board_quality", "connection reference"=w426) -> ("error out"=w407:errorcluster, "connection out"=w425:T29, "错误状态"=w398:bool)  [unwired: 4 in]
                n376 = call "时间延迟5"("error in (no error)"=w407, "Delay Time (s)"=0.1) -> ("error out"=w411:errorcluster)  [unwired: 9 in]
                n377 = case shown="真" w398 {
                  frame False {
                  }
                  frame True {
                    w431 = "" ("产品型号")
                    n378 = local write "产品型号"(w431) -> ()
                    n379 = local write "载具码"(w431) -> ()
                    n380 = local write "产品编码"(w431) -> ()
                  }
                }
                n381 = call "升立德IO读写Main.vi"("结果"=w398, "error in"=w411, "选项"=升立德IOAction."写成功/失败信号ON") -> ("error out"=w406:errorcluster)  [unwired: 4 in, 4 out]
                n382 = call "AddMsg.vi"("Result"=w398, "添加消息"="上传process数据", "消息Action"=MsgAction."区分结果添加消息") -> ()  [unwired: 1 in, 1 out]
              }
            }
          }
          n383 = call "相机1初始化.vi"() -> ("Session Out"=w104:T11, "Image"=w106:T3, "相机1状态"=w105:bool)  [unwired: 1 in, 1 out]
          n384 = while {
            shift-right: [w530] -> _
            shift-left: w105 -> [w527]
            shift-right: [w531] -> _
            shift-left: w104 -> [w528]
            shift-right: [w525] -> _
            shift-left: w106 -> [w526]
            tunnel: w94 -> [w521]
            stop <- w532 stop-if-true
            # "相机1处理程序"
            n385 = Dequeue Element(queue=w521, timeout in ms (-1)=5 ("超时毫秒(-1)")) -> (queue out=w524:refnum<queue>, element=w529:T24, error out=w523:errorcluster)  [unwired: 1 in, 1 out]
            n386 = case shown="\"Cam1自动:Mark2\"" w529 {
              tunnel: w528 -> [w536 w539 w546 w551 w554 w564 w574 w586 w596 w604 w608 w628]
              tunnel: [w536 w538 w545 w550 w554 w562 w571 w584 w594 w602 w619 w637] -> w531
              tunnel: w526 -> [w535 w540 w544 w549 w553 w563 w573 w585 w595 w603 w617 w638]
              tunnel: [w534 w541 w543 w548 w552 w561 w572 w583 w593 w601 w616 w624] -> w530
              tunnel: [w535 w540 w544 w549 w553 w557 w570 w582 w591 w599 w618 w636] -> w525
              tunnel: w527 -> [w534 w541 w543 w548 w552 _ _ _ _ _ _ _]
              tunnel: w524 -> [_ _ _ _ _ w560 w569 _ _ _ _ _]
              tunnel: w523 -> [_ _ _ _ _ _ _ _ _ _ _ _]
              tunnel: [TRUE ("Mark点拍照结果") _ _ _ _ TRUE ("Mark点拍照结果") TRUE ("Mark点拍照结果") TRUE ("Mark点拍照结果") TRUE ("Mark点拍照结果") TRUE ("Mark点拍照结果") w605 w625] -> w520
              frame "Cam1初始化" {
              }
              frame "Cam1更新曝光时间-拍Mark点1" {
                n387 = call "相机写曝光时间.vi"("选择相机和拍照对象"=控件-选择相机和拍照对象."相机1拍Mark1", "Session in"=w539) -> ("Session Out"=w538:T11)  [unwired: 9 in]
              }
              frame "Cam1更新曝光时间-拍Mark点2" {
                n388 = call "相机写曝光时间.vi"("选择相机和拍照对象"=控件-选择相机和拍照对象."相机1拍Mark2", "Session in"=w546) -> ("Session Out"=w545:T11)  [unwired: 9 in]
              }
              frame "Cam1更新曝光时间-拍照二维码" {
                n389 = call "相机写曝光时间.vi"("选择相机和拍照对象"=控件-选择相机和拍照对象."相机1拍二维码", "Session in"=w551) -> ("Session Out"=w550:T11)  [unwired: 9 in]
              }
              frame "Cam1待命", Default {
              }
              frame "Cam1实时-Mark" {
                n390 = call "相机1拍照.vi"("Image"=w563, "引用句柄输入"=w564) -> ("拍照结果"=w561:bool, "Image Out"=w558:T3, "引用句柄输出"=w562:T11, "取像时间"=w559:u32)  [unwired: 5 in, 1 out]
                n391 = local read "Cam1实时"() -> (w556:bool)
                n392 = case shown="真" w556 {
                  tunnel: w560 -> [_ w566]
                  frame False {
                  }
                  frame True {
                    n393 = Enqueue Element(queue=w566, element=Cam1QueueAction."Cam1实时-Mark" ("元素")) -> ()  [unwired: 2 in, 3 out]
                  }
                }
                n394 = call "显示取像时间-右下角.vi"("取像时间"=w559, "引用句柄输入"=w558) -> ("Image Out"=w557:T3)  [unwired: 9 in]
              }
              frame "Cam1实时-二维码" {
                n395 = local read "Cam1实时"() -> (w568:bool)
                n396 = call "相机1拍照.vi"("Image"=w573, "引用句柄输入"=w574) -> ("拍照结果"=w572:bool, "Image Out"=w575:T3, "引用句柄输出"=w571:T11, "取像时间"=w576:u32)  [unwired: 5 in, 1 out]
                n397 = case shown="真" w568 {
                  tunnel: w569 -> [_ w578]
                  frame False {
                  }
                  frame True {
                    n398 = Enqueue Element(queue=w578, element=Cam1QueueAction."Cam1待命" ("元素")) -> ()  [unwired: 2 in, 3 out]
                  }
                }
                n399 = call "显示取像时间-右下角.vi"("取像时间"=w576, "引用句柄输入"=w575) -> ("Image Out"=w570:T3)  [unwired: 9 in]
              }
              frame "Cam1手动:Mark1" {
                n400 = call "相机1拍照.vi"("切换曝光时间用Snap？"=TRUE, "Image"=w585, "引用句柄输入"=w586) -> ("拍照结果"=w583:bool, "Image Out"=w582:T3, "引用句柄输出"=w584:T11, "取像时间"=w580:u32)  [unwired: 4 in, 1 out]
                n401 = call "相机1-分析PCB孔影像-校准和自动共用.vi"("拍照功能"=控件-拍照PCB孔分类."拍照孔-Mark1" ("拍PCB孔功能"), "取像时间"=w580, "Image In"=w582) -> ()  [unwired: 3 in, 6 out]
              }
              frame "Cam1手动:Mark2" {
                # "手动时不更新良率"
                n402 = call "相机1拍照.vi"("切换曝光时间用Snap？"=TRUE, "Image"=w595, "引用句柄输入"=w596) -> ("拍照结果"=w593:bool, "Image Out"=w591:T3, "引用句柄输出"=w594:T11, "取像时间"=w592:u32)  [unwired: 4 in, 1 out]
                n403 = call "相机1-分析PCB孔影像-校准和自动共用.vi"("拍照功能"=控件-拍照PCB孔分类."拍照孔-Mark2", "取像时间"=w592, "Image In"=w591) -> ()  [unwired: 3 in, 6 out]
              }
              frame "Cam1手动:二维码" {
                n404 = call "相机1拍照.vi"("Image"=w603, "引用句柄输入"=w604) -> ("拍照结果"=w601:bool, "Image Out"=w599:T3, "引用句柄输出"=w602:T11, "取像时间"=w598:u32)  [unwired: 5 in, 1 out]
                n405 = call "相机1-分析PCB孔影像-校准和自动共用.vi"("拍照功能"=控件-拍照PCB孔分类."拍照二维码", "取像时间"=w598, "Image In"=w599) -> ()  [unwired: 3 in, 6 out]
              }
              frame "Cam1自动:Mark1" {
                (unwired) TRUE
                n406 = call "相机写曝光时间.vi"("选择相机和拍照对象"=控件-选择相机和拍照对象."相机1拍Mark1", "Session in"=w608) -> ("Session Out"=w607:T11)  [unwired: 9 in]
                n407 = disable-structure shown="禁用" {
                  frame Disabled {
                    n408 = local write "线号输入"(1 ("线号")) -> ()
                  }
                  frame Enabled {
                  }
                }
                n409 = call "相机1拍照.vi"("切换曝光时间用Snap？"=TRUE, "Image"=w617, "引用句柄输入"=w607) -> ("拍照结果"=w616:bool, "Image Out"=w618:T3, "引用句柄输出"=w619:T11, "取像时间"=w622:u32)  [unwired: 4 in, 1 out]
                n410 = call "升立德IO读写Main.vi"("选项"=升立德IOAction."写成功&&失败信号OFF") -> ("error out"=w614:errorcluster)  [unwired: 6 in, 4 out]
                n411 = call "相机1-分析PCB孔影像-校准和自动共用.vi"("error in (no error)"=w614, "拍照功能"=控件-拍照PCB孔分类."拍照孔-Mark1", "取像时间"=w622, "Image In"=w618) -> ("error out"=w612:errorcluster, "Mark点拍照结果"=w605:bool, "视觉补偿机械手移动量 mm"=→"mark1偏移":T13)  [unwired: 2 in, 3 out]
                n412 = call "时间延迟2"("error in (no error)"=w612, "Delay Time (s)"=0.1) -> ("error out"=w611:errorcluster)  [unwired: 9 in]
                n413 = call "升立德IO读写Main.vi"("结果"=w605, "error in"=w611, "选项"=升立德IOAction."写成功/失败信号ON") -> ()  [unwired: 4 in, 5 out]
              }
              frame "Cam1自动:Mark2" {
                (unwired) TRUE
                n414 = call "相机写曝光时间.vi"("选择相机和拍照对象"=控件-选择相机和拍照对象."相机1拍Mark2", "Session in"=w628) -> ("Session Out"=w627:T11)  [unwired: 9 in]
                n415 = call "相机1拍照.vi"("切换曝光时间用Snap？"=TRUE, "Image"=w638, "引用句柄输入"=w627) -> ("拍照结果"=w624:bool, "Image Out"=w636:T3, "引用句柄输出"=w637:T11, "取像时间"=w641:u32)  [unwired: 4 in, 1 out]
                n416 = call "升立德IO读写Main.vi"("选项"=升立德IOAction."写成功&&失败信号OFF") -> ("error out"=w633:errorcluster)  [unwired: 6 in, 4 out]
                n417 = call "相机1-分析PCB孔影像-校准和自动共用.vi"("error in (no error)"=w633, "拍照功能"=控件-拍照PCB孔分类."拍照孔-Mark2", "取像时间"=w641, "Image In"=w636) -> ("error out"=w632:errorcluster, "Mark点拍照结果"=w625:bool, "mark Angle"=→"mark Angle":sgl)  [unwired: 2 in, 3 out]
                n418 = case shown="真" w624 {
                  frame False {
                  }
                  frame True {
                    n419 = flat-sequence {
                      frame #0 {
                        n420 = local write "是否打开"(FALSE ("是否打开")) -> ()
                      }
                      frame #1 {
                        n421 = property on="打开表格" class="Bool (严格)"("Val(Sgnl)"=TRUE ("值(信号)")) -> ()  [unwired: 2 in, 2 out]
                      }
                    }
                  }
                }
                n422 = call "时间延迟"("error in (no error)"=w632, "Delay Time (s)"=0.1) -> ("error out"=w631:errorcluster)  [unwired: 9 in]
                n423 = call "升立德IO读写Main.vi"("结果"=w625, "error in"=w631, "选项"=升立德IOAction."写成功/失败信号ON") -> ()  [unwired: 4 in, 5 out]
              }
            }
            "上相机" <- w525
            "1#结果" <- w520
            n424 = local read "退出while"() -> (w532:bool)
            "相机1连线" <- w527
          }
          n425 = call <vilib>:"DB Tools Close Connection.vi"("error in (no error)"=w100, "connection reference"=w102) -> ("error out"=w99:errorcluster)  [unwired: 5 in]
          n426 = call <vilib>:"Clear Errors.vi"("error in (no error)"=w99) -> ()  [unwired: 5 in, 2 out]
          n427 = while {
            stop <- w516 stop-if-true
            # "只要相机就报警，就把整个背景变红色"
            n428 = local read "IO卡连接"() -> (w513:bool)
            n429 = local read "相机1连线"() -> (w515:bool)
            n430 = Wait (ms)(milliseconds to wait=u32 1000 ("等待时间（毫秒）")) -> ()  [unwired: 1 out]
            n431 = control-ref of="主控件"() -> (w514:refnum<vi>)
            n432 = Format Date/Time String(time format string (%c)="%H%M") -> (date/time string=w508:string)  [unwired: 2 in]
            n433 = Compound Arithmetic op=AND(w513, w515) -> ()  [unwired: 1 out]
            n434 = Decimal String To Number(string=w508) -> (number=w507:i32)  [unwired: 2 in, 1 out]
            n435 = In Range and Coerce(upper limit=1202 ("上限"), x=w507, lower limit=1200 ("下限")) -> (In Range?=w504:bool)  [unwired: 1 out]
            n436 = Select(t=u32 16777216, s=TRUE, f=u32 16711680) -> (s? t:f=w518:u32)
            n437 = property on="属性节点" class="TabCtl (严格)"(reference=w514, "FG Color"=w518) -> ()  [unwired: 1 in, 2 out]
            n438 = case shown="真" w504 {
              frame False {
              }
              frame True {
                n439 = call "硬盘剩余空间查询.vi"() -> ("磁盘剩余空间不够"=w519:bool)  [unwired: 7 in, 2 out]
                n440 = Quit LabVIEW(quit? (T)=w519) -> ()
              }
            }
            n441 = local read "退出while"() -> (w516:bool)
          }
          n442 = while {
            tunnel: w94 -> [w446]
            tunnel: w95 -> [w432]
            tunnel: w96 -> [w434]
            stop <- w453 stop-if-true
            n443 = call "升立德IO读写Main.vi"("选项"=升立德IOAction."读信号(16bit)") -> ("error out"=w448:errorcluster, "触发上升沿"=w447:T4, "IO输入"=w444:T6, "IO输出"=w450:T5)  [unwired: 6 in, 1 out]
            "IO输入" <- w444
            "触发上升沿" <- w447
            n444 = local read "退出while"() -> (w453:bool)
            n445 = Unbundle By Name(w447) -> ("3 触发扫码"=w433:bool, "2 布线完成触发"=w435:bool, "4 要线信号"=w436:bool, "0 触发拍照Mark1"=w437:bool, "1 触发拍照Mark2"=w438:bool)
            n446 = local write "IO输出"(w450) -> ()
            n447 = Wait (ms)(milliseconds to wait=u32 30 ("等待时间（毫秒）")) -> ()  [unwired: 1 out]
            n448 = Unbundle By Name(w444) -> ("6 PLC自动运行"=w443:bool)
            n449 = call "升立德IO读写Main.vi"("error in"=w448, "选项"=升立德IOAction."写生命信号") -> ()  [unwired: 5 in, 5 out]
            n450 = Or(x=w437, y=w438) -> (x .or. y?=w445:bool)
            n451 = case shown="真" w433 {
              tunnel: w434 -> [_ w480]
              tunnel: w432 -> [_ w476]
              frame False {
              }
              frame True {
                n452 = call "基恩士扫码枪.vi"() -> ("error out"=w477:errorcluster, "扫码内容"=w478:string, "扫码成功"=w475:bool)  [unwired: 9 in]
                "扫码状态" <- w475
                n453 = property on="载具码" class="Str"("Value"=w478) -> ()  [unwired: 2 in, 2 out]
                n454 = local write "写一笔轨迹"(FALSE ("布尔")) -> ()
                n455 = case shown="真" w475 {
                  tunnel: w480 -> [_ w488]
                  tunnel: w477 -> [_ w484]
                  tunnel: w476 -> [_ w483]
                  frame False {
                  }
                  frame True {
                    n456 = property on="单机运行" class="Bool (严格)"() -> ("Value"=w481:bool)  [unwired: 2 in, 2 out]
                    n457 = Select(t=cluster{"msg":string, "Data":variant} {"msg"="下载布线表文件", "Data"=variant} ("元素"), s=w481, f=cluster{"msg":string, "Data":variant} {"msg"="获取产品编码", "Data"=variant} ("元素")) -> (s? t:f=w487:cluster{"msg":string, "Data":variant})
                    n458 = Enqueue Element(queue=w488, element=w487, error in (no error)=w484) -> (error out=w482:errorcluster)  [unwired: 1 in, 2 out]
                    n459 = case shown="真" w481 {
                      tunnel: w483 -> [_ w492]
                      tunnel: w482 -> [_ w491]
                      frame False {
                      }
                      frame True {
                        n460 = local write "加工代码"("1" ("加工代码")) -> ()
                        n461 = Enqueue Element(queue=w492, element=欧姆龙PLC_Action."写加工信号" ("元素"), error in (no error)=w491) -> ()  [unwired: 1 in, 3 out]
                      }
                    }
                  }
                }
              }
            }
            n462 = case shown="真" w435 {
              tunnel: w434 -> [_ w467]
              frame False {
              }
              frame True {
                n463 = local read "基本信息"() -> (w466:T12)
                n464 = local read "布线索引"() -> (w464:i32)
                n465 = Unbundle By Name(w466) -> ("线总数"=w465:dbl)
                n466 = call "AddMsg.vi"("添加消息"="布线完成触发", "消息Action"=MsgAction."添加消息") -> ()  [unwired: 2 in, 1 out]
                n467 = Increment(x=w464) -> (x+1=w463:i32)
                n468 = Equal?(x=w463, y=w465) -> (x = y?=w462:bool)
                n469 = case shown="真" w462 {
                  tunnel: w467 -> [_ w472]
                  tunnel: w463 -> [_ _]
                  frame False {
                    n470 = local read "线号显示"() -> (w469:i32)
                    n471 = Increment(x=w469) -> (x+1=w468:i32)
                    n472 = local write "线号显示"(w468) -> ()
                    n473 = local write "线号输入"(w468) -> ()
                  }
                  frame True {
                    w471 = 1 ("当前布线线号")
                    n474 = local write "线号显示"(w471) -> ()
                    n475 = local write "线号输入"(w471) -> ()
                    n476 = local read "单机运行"() -> (w470:bool)
                    n477 = case shown="假" w470 {
                      tunnel: w472 -> [w473 _]
                      frame False {
                        n478 = Enqueue Element(queue=w473, element=cluster{"msg":string, "Data":variant} {"msg"="上传ProcessData", "Data"=variant} ("元素")) -> ()  [unwired: 2 in, 3 out]
                      }
                      frame True {
                      }
                    }
                  }
                }
                n479 = call "升立德IO读写Main.vi"("选项"=升立德IOAction."写成功&&失败信号OFF") -> ("error out"=w461:errorcluster)  [unwired: 6 in, 4 out]
                n480 = call "时间延迟3"("error in (no error)"=w461, "Delay Time (s)"=0.1) -> ("error out"=w459:errorcluster)  [unwired: 9 in]
                n481 = call "升立德IO读写Main.vi"("结果"=TRUE, "error in"=w459, "选项"=升立德IOAction."写成功/失败信号ON") -> ()  [unwired: 4 in, 5 out]
              }
            }
            n482 = case shown="真" w436 {
              tunnel: w432 -> [_ w497]
              frame False {
              }
              frame True {
                n483 = Enqueue Element(queue=w497, element=欧姆龙PLC_Action."写基本信息" ("元素")) -> ()  [unwired: 2 in, 3 out]
                n484 = local write "写一笔轨迹"(TRUE ("布尔")) -> ()
                n485 = call "AddMsg.vi"("添加消息"="要线触发", "消息Action"=MsgAction."添加消息") -> ()  [unwired: 2 in, 1 out]
              }
            }
            n486 = case shown="真" w445 {
              tunnel: w446 -> [_ w503]
              tunnel: w437 -> [_ w499]
              frame False {
              }
              frame True {
                n487 = Select(t=Cam1QueueAction."Cam1自动:Mark1" ("元素"), s=w499, f=Cam1QueueAction."Cam1自动:Mark2" ("元素")) -> (s? t:f=w502:T24)
                n488 = Enqueue Element(queue=w503, element=w502) -> ()  [unwired: 2 in, 3 out]
                n489 = call "升立德IO读写Main.vi"("选项"=升立德IOAction."开光源") -> ()  [unwired: 6 in, 5 out]
              }
            }
            n490 = Select(t=T20."Disabled and Grayed Out" ("禁用"), s=w443, f=T20."Enabled" ("禁用")) -> (s? t:f=w440:T20)
            n491 = property on="线号输入" class="DigNum (严格)"("DisabledEnum"=w440) -> (error out=w439:errorcluster)  [unwired: 2 in, 1 out]
            n492 = call <vilib>:"Clear Errors.vi"("error in (no error)"=w439) -> ()  [unwired: 5 in, 2 out]
          }
          n493 = while {
            tunnel: w95 -> [w110]
            tunnel: w96 -> [w109]
            shift-right: [w107] -> _
            shift-left: _ -> [w108]
            stop <- w114 stop-if-true
            # "plc"
            n494 = local read "退出while"() -> (w114:bool)
            n495 = Dequeue Element(queue=w110, timeout in ms (-1)=1000 ("超时毫秒(-1)")) -> (queue out=w111:refnum<queue>, element=w112:T23)  [unwired: 1 in, 2 out]
            n496 = case shown="\"写基本信息\"" w112 {
              tunnel: w111 -> [_ _ w138 w171 w183 w195 _ _ w237 _]
              tunnel: w109 -> [_ w129 _ _ _ _ _ _ _ _]
              tunnel: w108 -> [w115 w124 w137 w159 w173 w185 w203 w213 w231 w239]
              tunnel: [w115 w123 w137 w159 w173 w185 w203 w213 w231 w239] -> w107
              frame "初始化" {
                n497 = call "欧姆龙PLC通讯Main-UDP.vi"("欧姆龙PLC Action"=欧姆龙PLC_Action."初始化") -> ("错误out"=w118:errorcluster, "PLC连线成功"=w116:bool)  [unwired: 8 in, 1 out]
                n498 = Unbundle By Name(w118) -> ("status"=w117:bool)
                n499 = Not(x=w117) -> ()  [unwired: 1 out]
                n500 = local write "PLC通讯"(w116) -> ()
              }
              frame "读设备状态", Default {
                n501 = disable-structure shown="禁用" {
                  frame Disabled {
                    n502 = Wait (ms)(milliseconds to wait=u32 500 ("等待时间（毫秒）")) -> ()  [unwired: 1 out]
                  }
                  frame Enabled {
                  }
                }
                n503 = global read "Global.vi" "其它规格"() -> (w125:T7)
                n504 = Unbundle By Name(w125) -> ("其它勾选类规格.上传设备状态数据"=w122:bool)
                n505 = call "欧姆龙PLC通讯Main-UDP.vi"("欧姆龙PLC Action"=欧姆龙PLC_Action."读设备状态") -> ("解码成U16数组"=w123:u16[])  [unwired: 8 in, 2 out]
                n506 = Not Equal?(x=w123, y=w124) -> (x != y?=w121:bool[])
                n507 = And Array Elements(Boolean array=w121) -> (logical AND=w120:bool)
                n508 = And(x=w122, y=w120) -> (x .and. y?=w126:bool)
                n509 = case shown="真" w126 {
                  tunnel: w129 -> [_ w136]
                  tunnel: "上传statusData" ("table") -> [_ w133]
                  tunnel: w123 -> [_ w132]
                  frame False {
                  }
                  frame True {
                    n510 = Number To Decimal String(number=w132) -> (decimal integer string=w131:string[])  [unwired: 1 in]
                    n511 = To Variant(anything=w131) -> (Variant=w134:variant)
                    n512 = Bundle("table"=w133, "Variant"=w134) -> (w135:cluster{"table":string, "Variant":variant})  [unwired: 1 in]
                    n513 = Enqueue Element(queue=w136, element=w135) -> ()  [unwired: 2 in, 3 out]
                  }
                }
              }
              frame "写基本信息" {
                n514 = stacked-sequence {
                  tunnel: w138 -> [_ _ w152]
                  frame #0 {
                    n515 = call "升立德IO读写Main.vi"("选项"=升立德IOAction."写成功&&失败信号OFF") -> ()  [unwired: 6 in, 5 out]
                  }
                  frame #1 {
                    n516 = local read "布线前甩线"() -> (w147:string[][])
                    n517 = local read "线号显示"() -> (w141:i32)
                    n518 = local read "加工代码"() -> (w140:string)
                    n519 = Fract/Exp String To Number(string=w147, default (0 dbl)=3.0 ("默认(0 DBL)")) -> (number=w146:dbl[][])  [unwired: 2 in, 1 out]
                    n520 = Index Array(array=w146, index (col)=0 ("禁用的索引 (列)")) -> (element=w143:dbl[])  [unwired: 1 in]
                    n521 = Decimal String To Number(string=w140) -> ()  [unwired: 2 in, 2 out]
                    n522 = Search 1D Array(1D array=w143, element=w141) -> (index of element=w142:i32)  [unwired: 1 in]
                    "布线索引" <- w142
                    n523 = local read "基本信息"() -> (w148:T12)
                    n524 = call "基本信息解析.vi"("线号"=w142, "基本信息"=w148) -> ("添加的数组"=w149:dbl[])  [unwired: 9 in]
                    "基本信息写入" <- w149
                    n525 = call "欧姆龙PLC通讯Main-UDP.vi"("写入数据"=w149, "欧姆龙PLC Action"=欧姆龙PLC_Action."写基本信息") -> ()  [unwired: 7 in, 3 out]
                  }
                  frame #2 {
                    n526 = case shown="假" "写一笔轨迹" {
                      tunnel: w152 -> [_ w158]
                      frame False {
                        n527 = call "时间延迟4"("Delay Time (s)"=0.1) -> ("error out"=w154:errorcluster)  [unwired: 10 in]
                        n528 = call "升立德IO读写Main.vi"("结果"=TRUE, "error in"=w154, "选项"=升立德IOAction."写成功/失败信号ON") -> ()  [unwired: 4 in, 5 out]
                      }
                      frame True {
                        n529 = Enqueue Element(queue=w158, element=欧姆龙PLC_Action."写入进线前段点位" ("元素")) -> ()  [unwired: 2 in, 3 out]
                      }
                    }
                  }
                }
              }
              frame "写入进线前段点位" {
                n530 = local read "布线前甩线"() -> (w163:string[][])
                n531 = local read "布线索引"() -> (w164:i32)
                n532 = Fract/Exp String To Number(string=w163, default (0 dbl)=3.0 ("默认(0 DBL)")) -> (number=w162:dbl[][])  [unwired: 2 in, 1 out]
                n533 = Enqueue Element(queue=w171, element=欧姆龙PLC_Action."写入板内布线点位" ("元素")) -> ()  [unwired: 2 in, 3 out]
                n534 = local read "基本信息"() -> (w169:T12)
                n535 = Index Array(array=w162, index (row)=w164) -> (element=w160:dbl[])  [unwired: 1 in]
                n536 = call "plc传输点位补偿.vi"("选项"=enum16{"布线前甩线", "布线", "布线后甩线"}."布线前甩线", "基本信息"=w169, "行"=w164, "数组输入"=w160) -> ("数组输出"=w167:dbl[])  [unwired: 7 in]
                n537 = Array Subset(array=w167, index=1 ("索引")) -> (w165:dbl[])  [unwired: 1 in]
                n538 = call "欧姆龙PLC通讯Main-UDP.vi"("写入数据"=w165, "欧姆龙PLC Action"=欧姆龙PLC_Action."写入进线前段点位") -> ()  [unwired: 7 in, 3 out]
              }
              frame "写入板内布线点位" {
                n539 = local read "布线索引"() -> (w174:i32)
                n540 = local read "基本信息"() -> (w178:T12)
                n541 = local read "布线点位"() -> (w181:string[][])
                n542 = Enqueue Element(queue=w183, element=欧姆龙PLC_Action."写入出线布线点位" ("元素")) -> ()  [unwired: 2 in, 3 out]
                n543 = Fract/Exp String To Number(string=w181, default (0 dbl)=3.0 ("默认(0 DBL)")) -> (number=w179:dbl[][])  [unwired: 2 in, 1 out]
                n544 = Index Array(array=w179, index (row)=w174) -> (element=w177:dbl[])  [unwired: 1 in]
                n545 = call "plc传输点位补偿.vi"("选项"=enum16{"布线前甩线", "布线", "布线后甩线"}."布线", "基本信息"=w178, "行"=w174, "数组输入"=w177) -> ("数组输出"=w176:dbl[])  [unwired: 7 in]
                n546 = call "欧姆龙PLC通讯Main-UDP.vi"("写入数据"=w176, "欧姆龙PLC Action"=欧姆龙PLC_Action."写入板内布线点位") -> ()  [unwired: 7 in, 3 out]
              }
              frame "写入出线布线点位" {
                n547 = local read "布线后甩线"() -> (w199:string[][])
                n548 = local read "基本信息"() -> (w189:T12)
                n549 = local read "布线索引"() -> (w186:i32)
                n550 = Fract/Exp String To Number(string=w199, default (0 dbl)=3.0 ("默认(0 DBL)")) -> (number=w192:dbl[][])  [unwired: 2 in, 1 out]
                n551 = Enqueue Element(queue=w195, element=欧姆龙PLC_Action."写入进出线方向" ("元素")) -> ()  [unwired: 2 in, 3 out]
                n552 = Index Array(array=w192, index (row)=w186) -> (element=w191:dbl[])  [unwired: 1 in]
                n553 = call "plc传输点位补偿.vi"("选项"=enum16{"布线前甩线", "布线", "布线后甩线"}."布线后甩线", "基本信息"=w189, "行"=w186, "数组输入"=w191) -> ("数组输出"=w190:dbl[])  [unwired: 7 in]
                n554 = call "欧姆龙PLC通讯Main-UDP.vi"("写入数据"=w190, "欧姆龙PLC Action"=欧姆龙PLC_Action."写入出线布线点位") -> ()  [unwired: 7 in, 3 out]
                n555 = local read "布线前甩线"() -> (w201:string[][])
                n556 = local read "布线点位"() -> (w200:string[][])
                n557 = local read "基本信息"() -> (w197:T12)
                n558 = Bundle By Name(cluster=w197, "序号"=w186) -> (w187:T12)
                n559 = call "布线趋势图示-单根.vi"("基本信息"=w187, "布线前甩线"=w201, "布线点位"=w200, "布线后甩线"=w199, "轨迹选择"="轨迹选择") -> ("引用句柄输出"=w198:T3)  [unwired: 14 in]
                n560 = local write "当前线号布线轨迹示意图"(w198) -> ()
                n561 = local write "基本信息"(w187) -> ()
              }
              frame "写入数据写入完成信号" {
                n562 = local read "线号显示"() -> (w210:i32)
                n563 = call "升立德IO读写Main.vi"("结果"=TRUE, "选项"=升立德IOAction."写成功/失败信号ON") -> ()  [unwired: 5 in, 5 out]
                n564 = Number To Decimal String(number=w210) -> (decimal integer string=w208:string)  [unwired: 1 in]
                n565 = Concatenate Strings("写入PLC线号" ("消息显示"), w208, "完成" ("字符串")) -> (w206:string)
                n566 = call "AddMsg.vi"("Result"=TRUE, "添加消息"=w206, "消息Action"=MsgAction."添加消息") -> ()  [unwired: 1 in, 1 out]
              }
              frame "获取信息" {
                n567 = local read "布线前甩线"() -> (w216:string[][])
                n568 = local read "线号显示"() -> (w215:i32)
                n569 = Fract/Exp String To Number(string=w216, default (0 dbl)=3.0 ("默认(0 DBL)")) -> (number=w217:dbl[][])  [unwired: 2 in, 1 out]
                n570 = Index Array(array=w217, index (col)=0 ("禁用的索引 (列)")) -> (element=w220:dbl[])  [unwired: 1 in]
                n571 = Search 1D Array(1D array=w220, element=w215) -> (index of element=w214:i32)  [unwired: 1 in]
                n572 = local read "布线前甩线"() -> (w221:string[][])
                n573 = local read "布线后甩线"() -> (w225:string[][])
                n574 = local read "基本信息"() -> (w229:T12)
                n575 = local read "布线点位"() -> (w226:string[][])
                n576 = Bundle By Name(cluster=w229, "序号"=w214) -> (w228:T12)
                n577 = local read "轨迹选择"() -> (w227:u16)
                n578 = call "布线趋势图示-单根.vi"("基本信息"=w228, "布线前甩线"=w221, "布线点位"=w226, "布线后甩线"=w225, "轨迹选择"=w227) -> ("引用句柄输出"=→"当前线号布线轨迹示意图":T3)  [unwired: 14 in]
                n579 = call "AddMsg.vi"("Result"=TRUE, "添加消息"="手动展示轨迹" ("消息显示"), "消息Action"=MsgAction."添加消息") -> ()  [unwired: 1 in, 1 out]
              }
              frame "写入进出线方向" {
                n580 = local read "进出线编码"() -> (w235:cluster{"进线编码":i32, "出线编码":i32}[])
                n581 = local read "布线索引"() -> (w232:i32)
                n582 = Index Array(array=w235, index=w232) -> (element=w234:cluster{"进线编码":i32, "出线编码":i32})
                n583 = Enqueue Element(queue=w237, element=欧姆龙PLC_Action."写入数据写入完成信号" ("元素")) -> ()  [unwired: 2 in, 3 out]
                n584 = Cluster To Array(cluster=w234) -> (array=w233:i32[])
                n585 = call "欧姆龙PLC通讯Main-UDP.vi"("写入数据"=w233, "欧姆龙PLC Action"=欧姆龙PLC_Action."写入进出线方向") -> ()  [unwired: 7 in, 3 out]
              }
              frame "写加工信号" {
                n586 = stacked-sequence {
                  frame #0 {
                    n587 = call "升立德IO读写Main.vi"("选项"=升立德IOAction."写成功&&失败信号OFF") -> ()  [unwired: 6 in, 5 out]
                  }
                  frame #1 {
                    n588 = local read "加工代码"() -> (w243:string)
                    n589 = Decimal String To Number(string=w243) -> (number=w242:i32)  [unwired: 2 in, 1 out]
                    n590 = Build Array(w242) -> (w241:i32[])
                    n591 = call "欧姆龙PLC通讯Main-UDP.vi"("写入数据"=w241, "欧姆龙PLC Action"=欧姆龙PLC_Action."写加工信号") -> ()  [unwired: 7 in, 3 out]
                  }
                  frame #2 {
                    n592 = call "时间延迟6"("Delay Time (s)"=0.1) -> ("error out"=w246:errorcluster)  [unwired: 10 in]
                    n593 = call "升立德IO读写Main.vi"("结果"=TRUE, "error in"=w246, "选项"=升立德IOAction."写成功/失败信号ON") -> ()  [unwired: 4 in, 5 out]
                  }
                }
              }
            }
          }
        }
        frame #2 {
          # "这里可以关闭卡 等等..........."
          n594 = local read "退出Labview"() -> (w881:bool)
          n595 = case shown="真" w881 {
            frame False {
            }
            frame True {
              n596 = Quit LabVIEW(quit? (T)=TRUE ("退出？(T)")) -> ()
            }
          }
        }
      }
      n597 = disable-structure shown="禁用" {
        frame Disabled {
          n598 = call "线号.vi"() -> ()  [unwired: 11 in, 1 out]
        }
        frame Enabled {
        }
      }
    }
  }
  n599 = disable-structure shown="禁用" {
    frame Disabled {
      n600 = call "读取生产统计数据.vi"() -> (2:w883)  [unwired: 8 in, 1 out]
      n601 = local write item#-1(w883) -> ()
    }
    frame Enabled {
    }
  }
  n602 = disable-structure shown="禁用" {
    frame Disabled {
      n603 = call "根据规格存OKNG图存数据到缓存.vi"() -> ()  [unwired: 12 in]
      n604 = call "生产统计数据Main.vi"() -> ()  [unwired: 6 in, 4 out]
      n605 = call "欧姆龙PLC通讯Main-UDP.vi"() -> ()  [unwired: 9 in, 3 out]
      n606 = call "计算相机1补偿量.vi"() -> ()  [unwired: 7 in, 5 out]
      n607 = call "Main-数据保存.vi"() -> ()  [unwired: 9 in, 1 out]
    }
    frame Enabled {
    }
  }
  n608 = disable-structure shown="禁用" {
    frame Disabled {
      n609 = call "读触发信息-触发不同拍照流程.vi"() -> ("7触发上位机读锁附结果"=w884:bool)  [unwired: 10 in, 1 out]
      n610 = call "Main-数据保存.vi"() -> ()  [unwired: 9 in, 1 out]
      n611 = call "升立德IO读写Main.vi"() -> ()  [unwired: 7 in, 5 out]
      n612 = Or(y=w884) -> ()  [unwired: 1 in, 1 out]
    }
    frame Enabled {
    }
  }
  n613 = disable-structure shown="启用" {
    frame Disabled {
      n614 = global read "Global.vi" "已输入密码"() -> (w885:bool)
      n615 = case shown="真" {
        selector: _ -> [_ _]
        tunnel: _ -> [_ w892]
        frame False {
        }
        frame True {
          n616 = local read "当前零件序号"() -> (w896:i32)
          n617 = call "ModeEditMain.vi"("当前零件序号"=w896) -> ("ModelEditInfo"=w890:T1, "产品程式设定OK"=w888:bool)
          n618 = Unbundle By Name(w890) -> ("点位信息表"=w889:string[][], "所有零件型号"=w894:string[], "当前零件序号"=w893:i32, "当前零件型号"=w895:string)
          n619 = global write "Global.vi" "ModelEditInfo"(w890) -> ()
          n620 = local write item#-1(w888) -> ()
          n621 = local write "点位信息表"(w889) -> ()
          n622 = property on="选择产品型号" class="Ring (严格)"("Strings []"=w894, "Value"=w893) -> ()  [unwired: 2 in, 2 out]
          n623 = local write "当前零件序号"(w893) -> ()
          n624 = local write "当前零件型号"(w895) -> ()
          n625 = call "读取生产统计数据.vi"("产品码"=w895) -> (2:w891)  [unwired: 7 in, 1 out]
          n626 = disable-structure shown="禁用" {
            frame Disabled {
              n627 = global write "Global.vi" "已输入密码"(TRUE ("已输入密码")) -> ()
            }
            frame Enabled {
            }
          }
          n628 = local write item#-1(w891) -> ()
          n629 = flat-sequence {
            tunnel: w892 -> [w900]
            tunnel: w890 -> [_]
            tunnel: w888 -> [w899]
            frame #0 {
              n630 = Unbundle By Name(w900) -> ("Cam1队列"=w904)
              n631 = control-ref of="当前线号布线轨迹示意图"() -> (w901:refnum<vi>)
              n632 = Enqueue Element(queue=w904, element=Cam1QueueAction."Cam1更新曝光时间-拍Mark点1" ("元素")) -> (error out=w903:errorcluster)  [unwired: 2 in, 2 out]
              n633 = call <vilib>:"Clear Errors.vi"("error in (no error)"=w903) -> ()  [unwired: 5 in, 2 out]
              n634 = call "下发产品测试信息给PLC.vi"() -> ()  [unwired: 11 in, 1 out]
              n635 = call "显示所有PCB所有点位锁附信息.vi"("产品程式设定OK"=w899, "Img引用-实际点位"=w901, "显示点位动作"=控件-显示锁附结果动作."初始化锁附结果示意图") -> ()  [unwired: 8 in, 1 out]
            }
          }
        }
      }
      n636 = case shown="假" w885 {
        tunnel: [w886 TRUE ("密码正确")] -> _
        frame False {
          n637 = call "输入密码对话框.vi"() -> ("密码正确"=w886:bool)  [unwired: 11 in]
        }
        frame True {
        }
      }
    }
    frame Enabled {
    }
  }
